vi "SubPanel_DataCollection_Rev11_v17.vi"(0 "DCPowerInformationClusterArray_Input":T1[](array[typedef]), 1 "VISAPowerInfoInputArray":T4[](array[typedef]), 2 "Run Data SubPanel Input":T6, 3 "RF Block Input Array":T5[](array[typedef]), 4 "Oscilloscope Configuration Input Array":T2[](array[typedef]) {"vertical coupling" items=["AC", "DC", "Ground"]}, 5 "Plot Color Array":u32[](array[colorbox])=[16711686, 65351, 8978420, 14474240, 16139007, 16752640, 8958719, 16758973, 16777215, 46792, 11992992, 12961221, 16763690, 12600063, 16711835, 2953983, 40796, 13111296, 13352613, 9221011, 12964076, 12819897, 65442, 16776704, 14540253, 16740729, 10658047, 10813344, 16753521, 13413843, 8691115, 10339240, 14401205, 16746704, 7467519, 16775978, 13872558, 11387603, 13354405, 10420227, 13107364, 4060, 35208, 11817216, 7566080, 40796, 7539456, 2837073, 6372186, 7499083, 10648702, 16757152], 6 "New Run?":bool, 7 "error in":errorcluster) -> (20 "DCPowerInformationClusterArray_Output":T1[](array[typedef]), 21 "VISAPowerInfoOutputArray":T4[](array[typedef]), 22 "Run Data SubPanel Output":T6, 23 "RF Subpanel Output":T5[](array[typedef]), 24 "Oscilloscope Info Array":T7(array[cluster]) {"vertical coupling" items=["AC", "DC", "Ground"]}, 25 "Reinitialize?":bool, 26 "Data Was Collected?":bool, 27 "error out":errorcluster)   [LabVIEW 2019]
uses:
  Controls/DataBlockControl.ctl
  Controls/RFBlockControl.ctl
  <instrlib>/niScope/Controls/niScope vertical coupling.ctl
  Controls/VISA_power_Control.ctl
  Controls/OscilloscopeBlockControl2.ctl
  Controls/DCPowerBlock_byInstrument_Control.ctl
  Controls/QueueDataControl_V3.ctl
  <instrlib>/niDMM/nidmm.llb/niDMM Trigger.ctl
  <instrlib>/niDMM/nidmm.llb/niDMM Resolution in Digits.ctl
  <instrlib>/niDMM/nidmm.llb/niDMM Function.ctl
  <instrlib>/niScope/Acquire/Fetch/niScope Multi Fetch Binary 16.vi
  <instrlib>/niDMM/nidmm.llb/niDMM Configure Measurement Digits.vi
  <vilib>/Utility/file.llb/Write Delimited Spreadsheet (string).vi
panel:
  out "error IO":errorcluster
  in  "Software Mitigation?":bool
  in  "User Forced Reset":bool
  in  "Total Time X Min":dbl
  in  "Total Time X Max":dbl
  in  "Total Current Y Min":dbl
  in  "Total Current Y Max":dbl
  in  "Total Voltage Y Min":dbl
  in  "Total Voltage Y Max":dbl
  in  "Total Measurement Range Update":bool
  in  "Live Measurement Range Update":bool
  in  "Live Current Y Min":dbl
  in  "Live Current Y Max":dbl
  in  "Live Voltage Y Min":dbl
  in  "Live Voltage Y Max":dbl
  in  "Waveform Update":bool
  in  "Current Waveform Y Max":dbl
  in  "Current Waveform Y Min":dbl
  in  "Voltage Waveform Y Min":dbl
  in  "Voltage Waveform Y Max":dbl
  in  "Max Range 7":dbl
  in  "Min Range 7":dbl
  in  "Min Range 6":dbl
  in  "Max Range 6":dbl
  in  "Max Range 5":dbl
  in  "Min Range 5":dbl
  in  "Max Range 4":dbl
  in  "Min Range 4":dbl
  in  "Min Range 3":dbl
  in  "Max Range 3":dbl
  in  "Min Range 2":dbl
  in  "Max Range 2":dbl
  in  "Min Range 0":dbl
  in  "Min Range 1":dbl
  in  "Max Range 1":dbl
  in  "Max Range 0":dbl
  in  "Oscope Range Update":bool
  out "Oscilloscope Configuration":T2 {"vertical coupling" items=["AC", "DC", "Ground"]}
  in  "Reset Value":i32=51
  out "Pryor's Graph":dbl[][](graph)
  in  "Reset Value 2":i32=251
  out "Channel Graph 0":dbl[](graph)
  out "Channel Graph 1":dbl[](graph)
  out "Channel Graph 2":dbl[](graph)
  out "Channel Graph 3":dbl[](graph)
  out "Channel Graph 7":dbl[](graph)
  out "Channel Graph 6":dbl[](graph)
  out "Channel Graph 5":dbl[](graph)
  out "Channel Graph 4":dbl[](graph)
  out "Measurement":dbl caption="BEAM STATE (NOT ~0 IF ON)" format="%.5f"
  in  "Time showing on Live Measurements":i32=251
  in  "Device Powered?":bool=TRUE
  out "Current Measurements Live":cluster{dbl[], dbl[]}[](graph)
  out "Voltage Measurements Live":cluster{dbl[], dbl[]}[](graph)
  out "Voltage Waveform Array":waveform(dbl)[](graph)
  out "Current Waveform Array":waveform(dbl)[](graph)
  out "Current Measurements Total":cluster{dbl[], dbl[]}[](graph)
  out "Voltage Measurements Total":cluster{dbl[], dbl[]}[](graph)
  out "Exiting":bool
  out "Full Run Information":string
  out "Ready For Next Run?":bool
  in  "Next Run":bool
  out "Recording Data":bool
  in  "Record Data Toggle":bool
  out "error of collection":errorcluster
  in  "force exit SubVI":bool
  out "RF Block Parameters Output":T5
  out "RFSourceInfoArray":string[][](array[string])
  out "OscilloscopeInfoArray":string[][](array[string])
  out "DCPowerInfoArray":string[][](array[string])
  # "Background information (Important)\nThere are three sets of voltage/current graphs\n\nOne is live always and just shows what all the channels look like _______ Waveform Array\n\nOne is live when measuring and shows some duration of the recording _______ Measurements Live\n\nOne shows the entire duration of the run, but it will take a few seconds to compile, just be patient it will populate\n\n\nInstructions (More Important)"
  # "CURRENTLY CAN ONLY USE ONE OSCOPE AT A TIME"
  # "off"
  # "on"
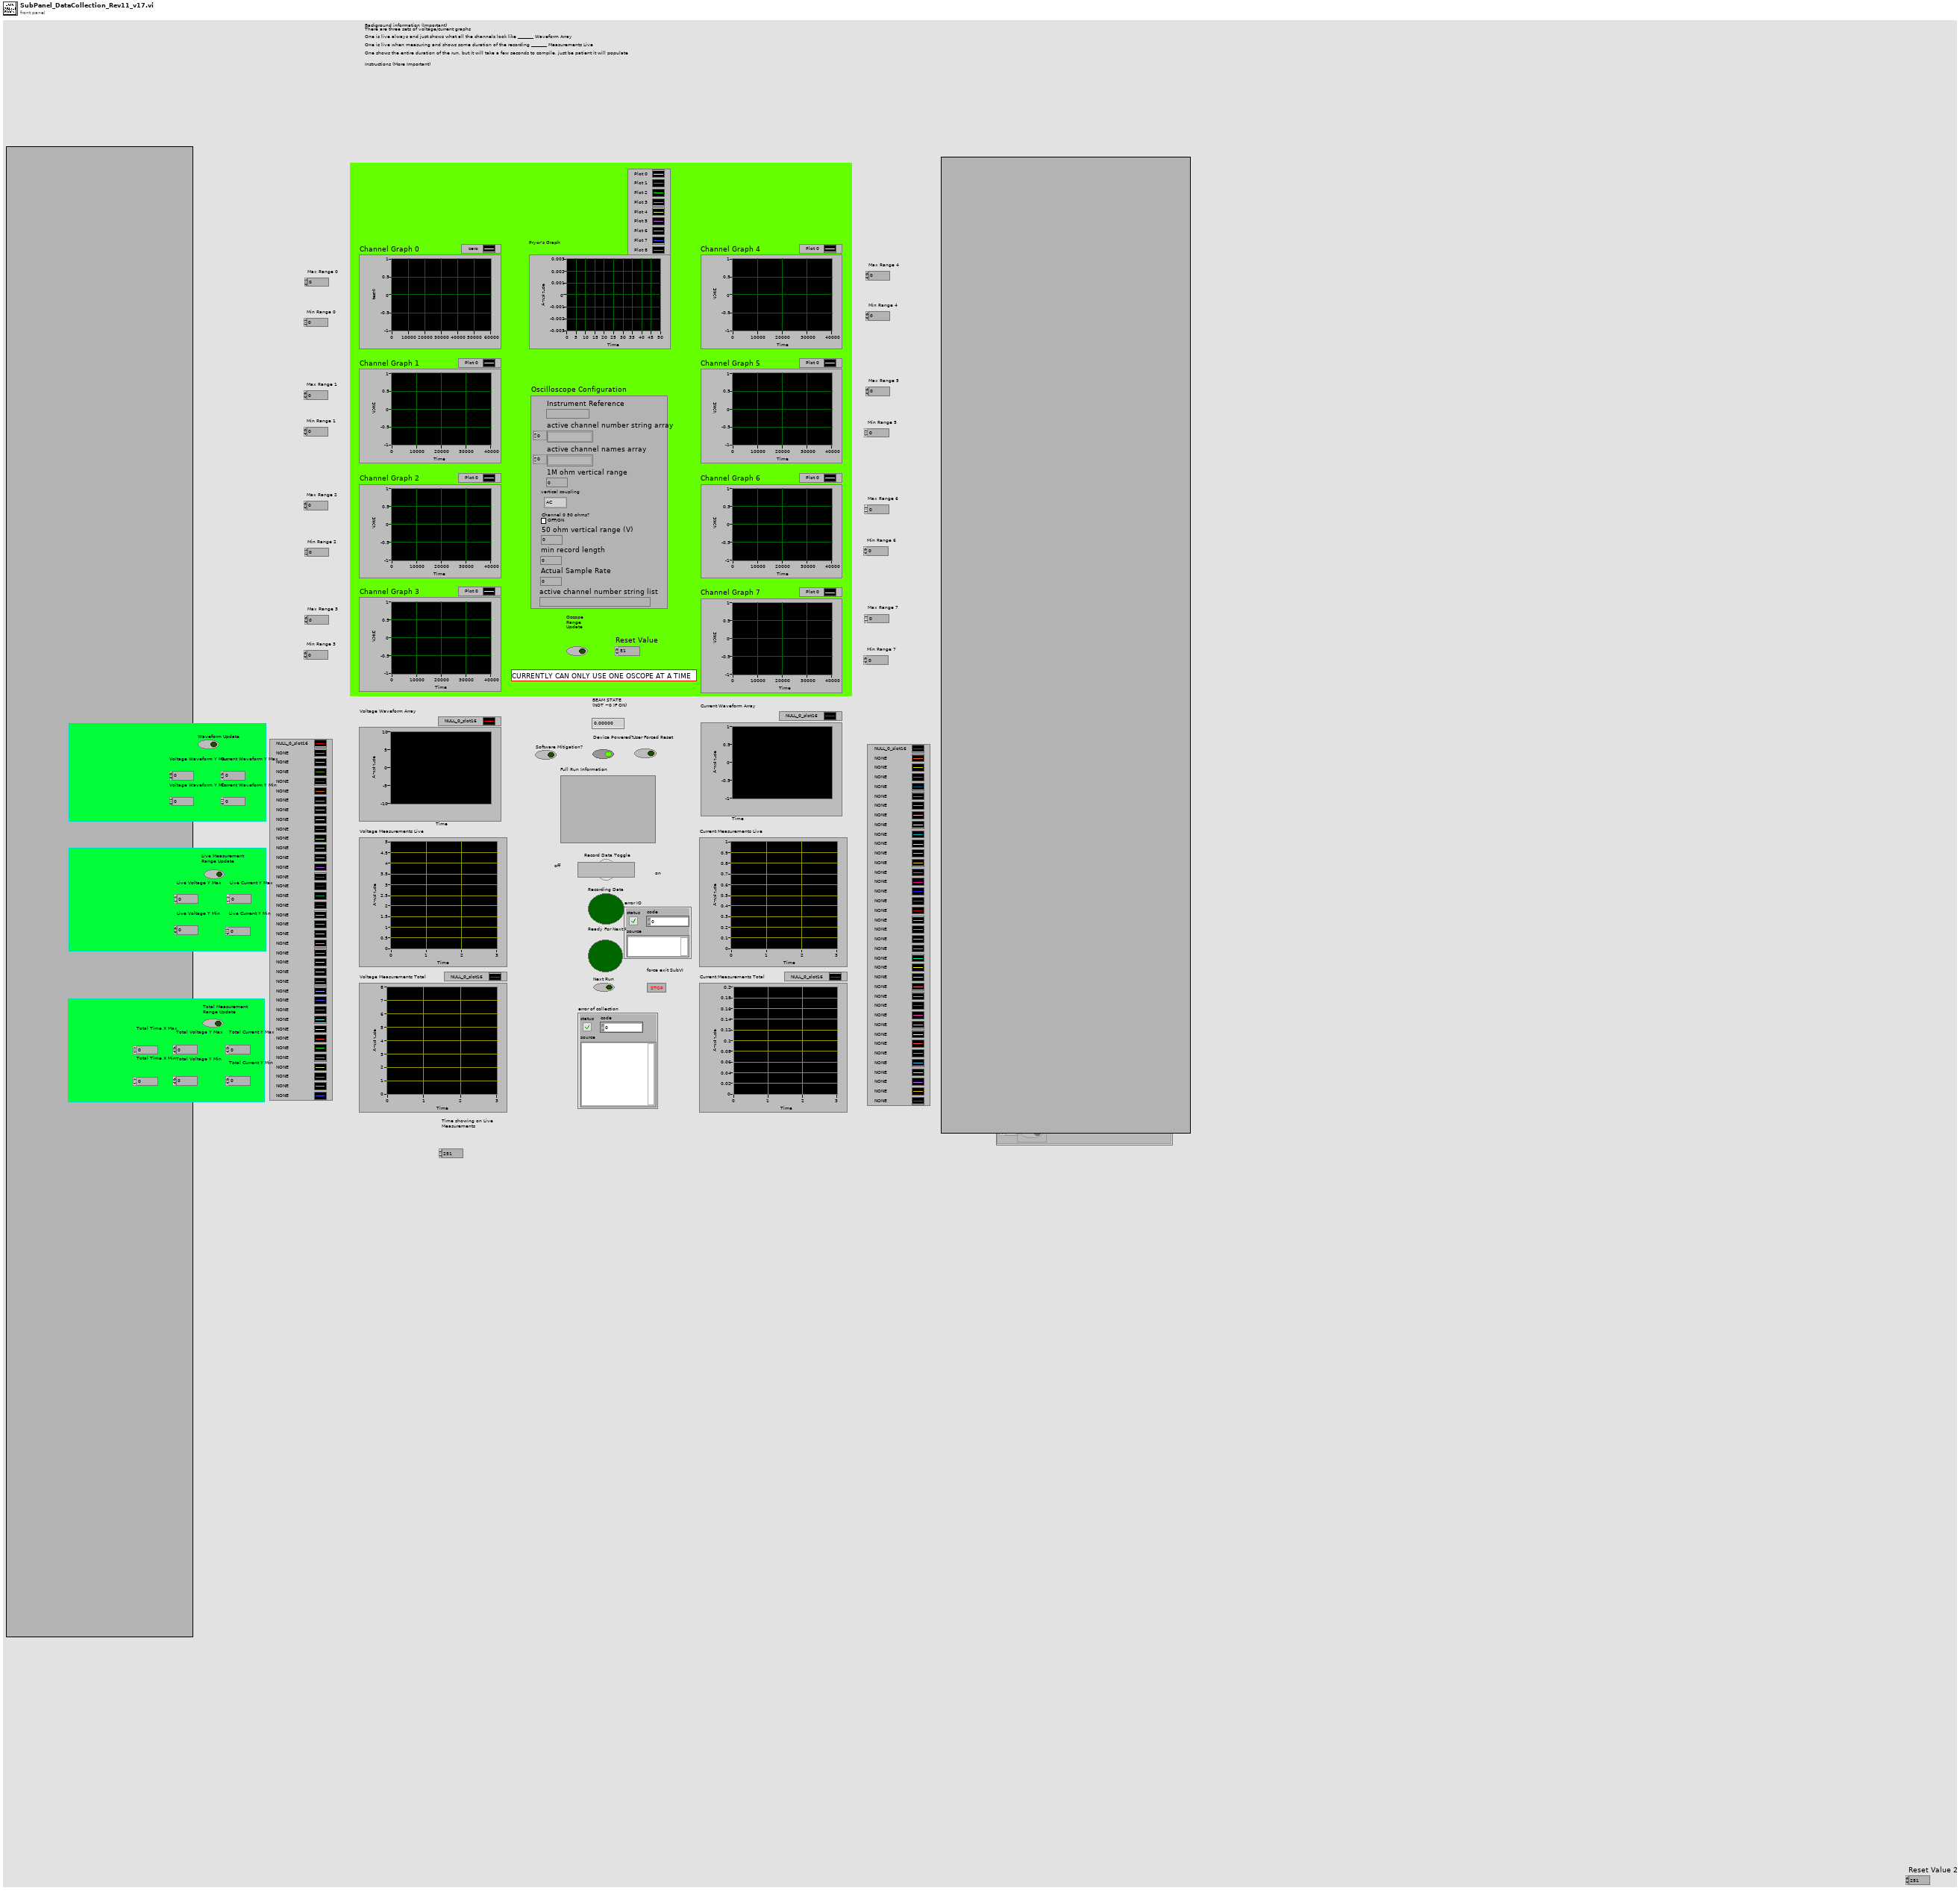
[diagram p1: front panel]
types:
  T1 = typedef "DCPowerBlock_byInstrument_Control.ctl" = cluster{"IVI Refnum out":refnum<k15>, "Active Channel Numbers String List":string, "Active Channel Numbers Array":string[], "Active Channel Voltage Array":dbl[], "Active Channel Names Array":string[], "Active Channel Current Limit Array":dbl[], "Active Channel Measure Record Delta Time Array":dbl[], "All Channel Numbers Array":string[], "Current Threshold Reset Value Array":dbl[], "Mitigation channel":bool[]}
  T2 = typedef "OscilloscopeBlockControl2.ctl" = cluster{"Instrument Reference":refnum<k15>, "active channel number string array":string[], "active channel names array":string[], "1M ohm vertical range":dbl, "vertical coupling":T3, "Channel 0 50 ohms?":bool, "50 ohm vertical range (V)":dbl, "min record length":i32, "Actual Sample Rate":dbl, "active channel number string list":string}
  T3 = typedef "niScope vertical coupling.ctl" = i32
  T4 = typedef "VISA_power_Control.ctl" = cluster{"VISA resource name":refnum<visa-resource-name>, "Active Channel List":string, "Active Channel Array":string[], "Input Array (Voltage,Current_Limit)":dbl[], "Input Array (Voltage,Current_Limit)":dbl[], "Channel Names":string[], "read buffer":string, "Channel Names Array":string[]}
  T5 = typedef "RFBlockControl.ctl" = cluster{"VISA resource name":refnum<visa-resource-name>, "RF Power State In":bool, "Frequency (GHz) Output":dbl, "Power (dBm) Output":dbl, "Instrument Name":string}
  T6 = typedef "DataBlockControl.ctl" = cluster{"Run Folder Parent Directory":path, "DUT":string, "Ion (ex Kr)":string, "Board Number":string, "Effective LET":string, "Test Type":enum16{"Single Event Latchup", "Single Event Transient", "Single Event Upset"}}
  T7 = cluster{"instrument handle out":refnum<k15>, string[], string[], "vertical range":dbl, "vertical coupling":T3, "Channel 0 50 ohms?":bool, "50 ohm vertical range (V)":dbl, "min record length":i32, "Actual Sample Rate":dbl, "channel names list":string}[]
  T8 = enum16{"open", "replace", "create", "open or create", "replace or create", "replace or create with confirmation"}
  T9 = cluster{"Array":dbl[], "Array":dbl[], "Array":dbl[], "Array":dbl[], "Array":dbl[], "Array":dbl[], "Array":dbl[], "Array":dbl[]}
  T10 = cluster{"wfm info":cluster{"actualSamples":i32, "absoluteInitialX":dbl, "relativeInitialX":dbl, "xIncrement":dbl, "offset":dbl, "gain":dbl, "reserved1":dbl, "reserved2":dbl}[], "wfm":i16[][]}
  T11 = typedef "niDMM Function.ctl" = enum16{"DC Volts", "AC Volts", "DC Current", "AC Current", "2-wire Resistance", "4-wire Resistance", "Diode", "Frequency", "Period", "AC Volts DC Coupled", "Capacitance", "Inductance", "Temperature"}
  T12 = typedef "niDMM Resolution in Digits.ctl" = dbl
  T13 = typedef "niDMM Trigger.ctl" = enum16{"Immediate", "External", "TTL 0", "TTL 1", "TTL 2", "TTL 3", "TTL 4", "TTL 5", "TTL 6", "Software", "TTL 7", "PXI Star", "LBR Trig 1", "Aux Trig 1"}
  T14 = cluster{"appended path":path, "refnum out":refnum<file>, "refnum out":refnum<file>, "refnum out":refnum<file>}
  T15 = typedef "QueueDataControl_V3.ctl" = cluster{"Array of fetched data":dbl[][][], "Channel Names Array":string[], "Voltage Waveform Array":waveform(dbl)[], "Current Waveform Array":waveform(dbl)[], "Resetting Time":timestamp, "Beam Logic":dbl}
  T16 = cluster{"IVI Refnum out":refnum<k15>, string, "voltage level channel 23":dbl, "Channel Name 23":string, "Current Limit":dbl, "Measure Record dt":dbl, string, "Current Threshold Reset Value Array":dbl, "Mitigation Channel":bool}[]
  T17 = cluster{"created path":path, refnum<file>[], refnum<file>[]}
  T18 = cluster{"created path":path, "DCPowerInformationArrayOutput_byChannel":cluster{"IVI Refnum out":refnum<k15>, string, "voltage level channel 23":dbl, "Channel Name 23":string, "Current Limit":dbl, "Measure Record dt":dbl, string, "Current Threshold Reset Value Array":dbl, "Mitigation Channel":bool}[], string[]}
  T19 = cluster{"actualSamples":i32, "absoluteInitialX":dbl, "relativeInitialX":dbl, "xIncrement":dbl, "offset":dbl, "gain":dbl, "reserved1":dbl, "reserved2":dbl}[]
  T20 = enum16{"big-endian, network order", "native, host order", "little-endian"}
  T21 = cluster{"Array of fetched data":dbl[][], string, i32[]}
  T22 = enum16{"Single Event Latchup", "Single Event Transient", "Single Event Upset"}
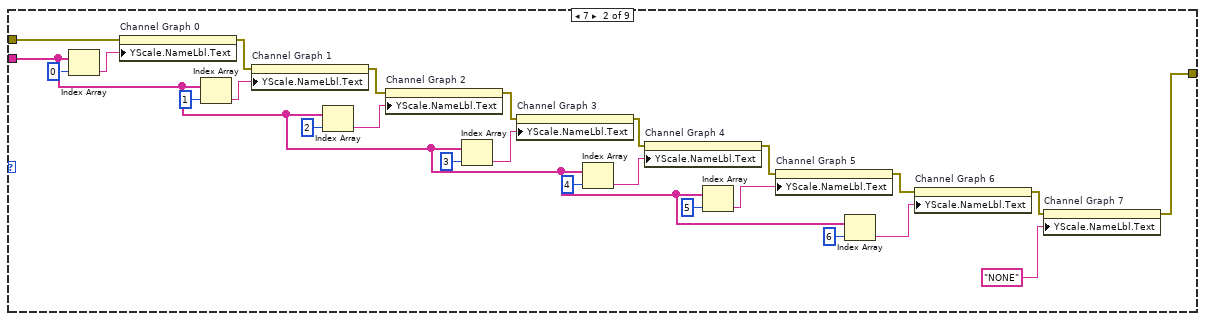
[diagram p2: hidden frame]
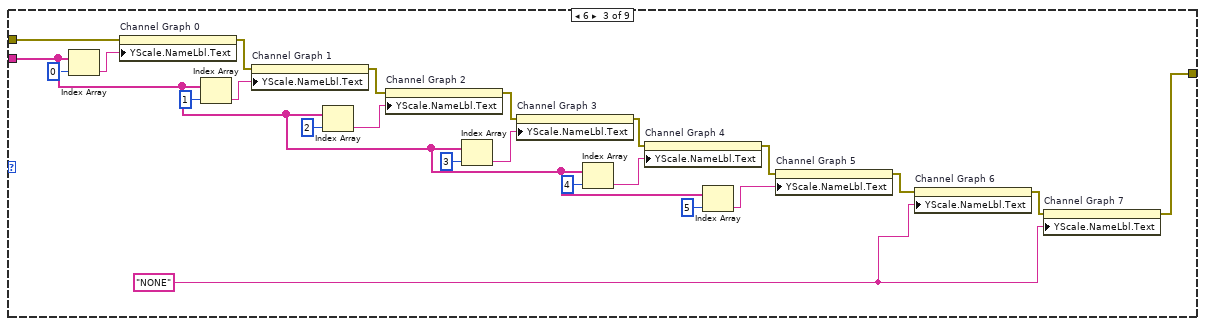
[diagram p3: hidden frame]
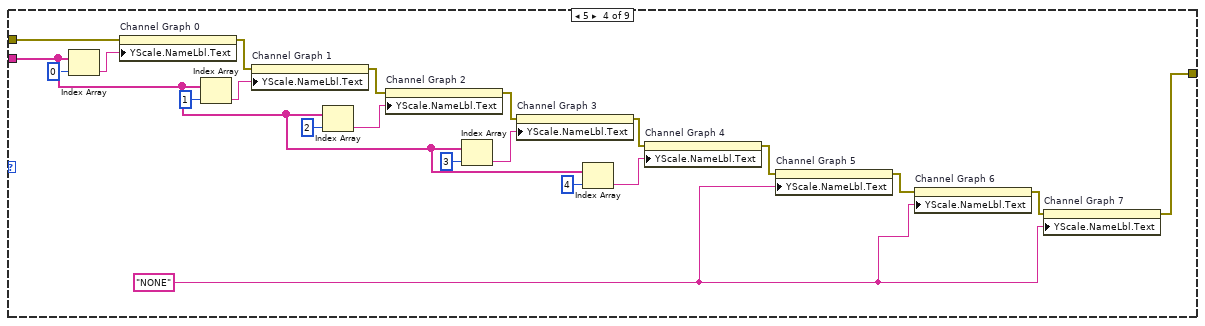
[diagram p4: hidden frame]
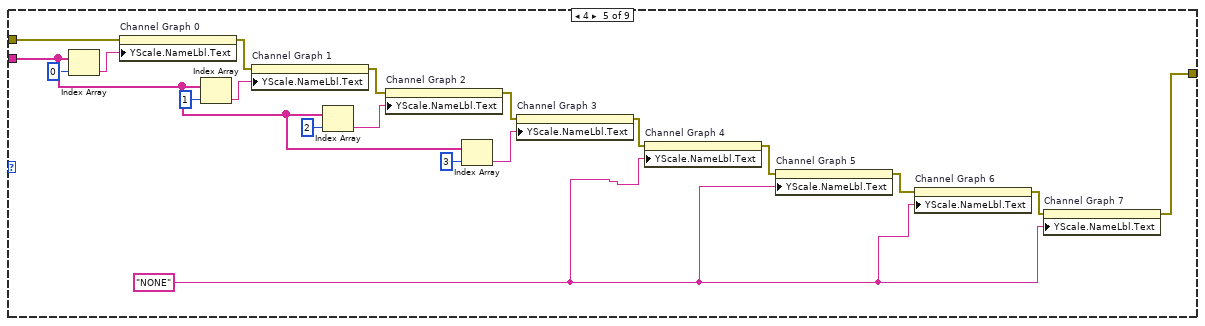
[diagram p5: hidden frame]
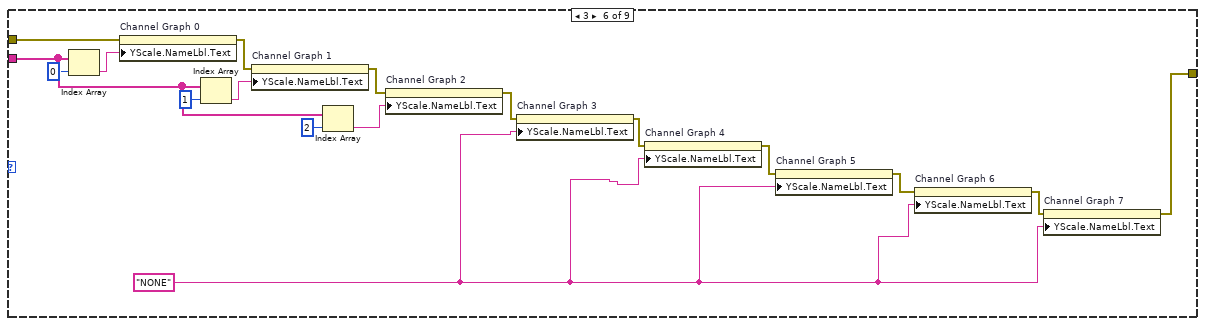
[diagram p6: hidden frame]
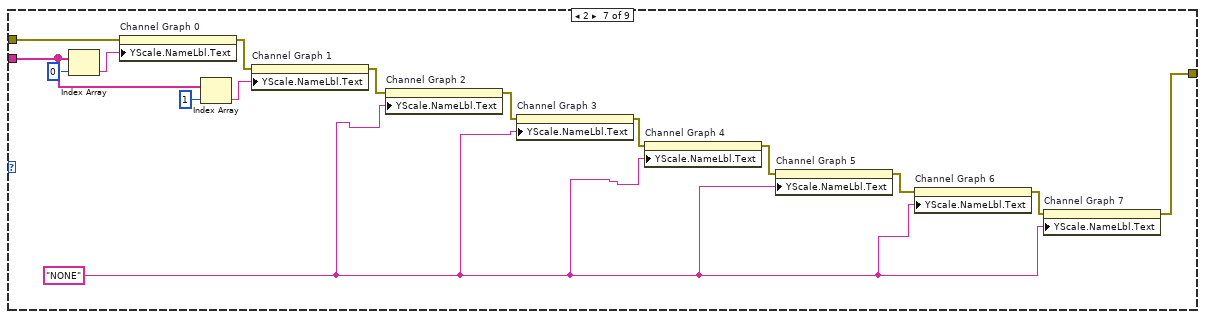
[diagram p7: hidden frame]
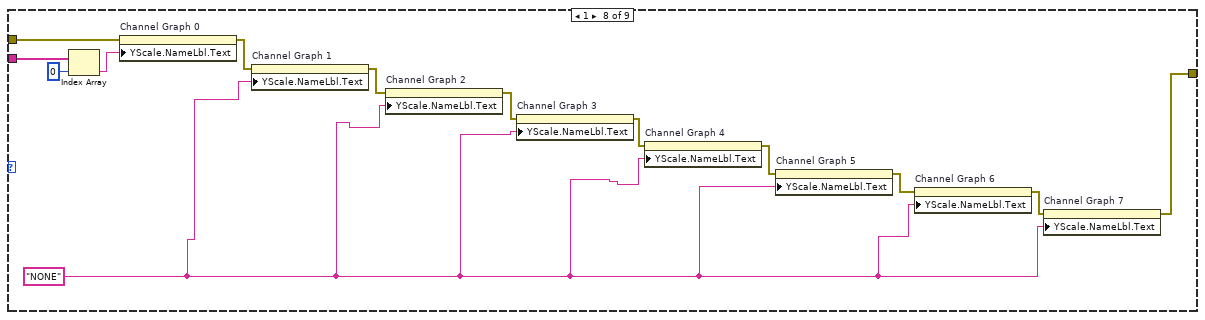
[diagram p8: hidden frame]
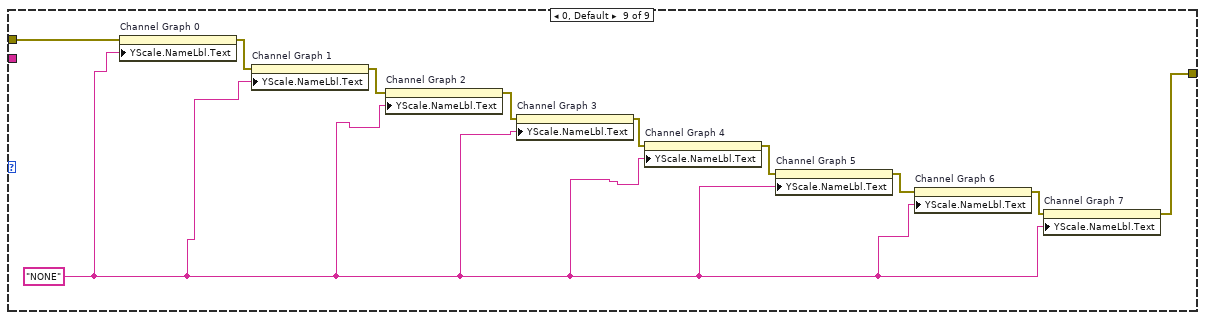
[diagram p9: hidden frame]
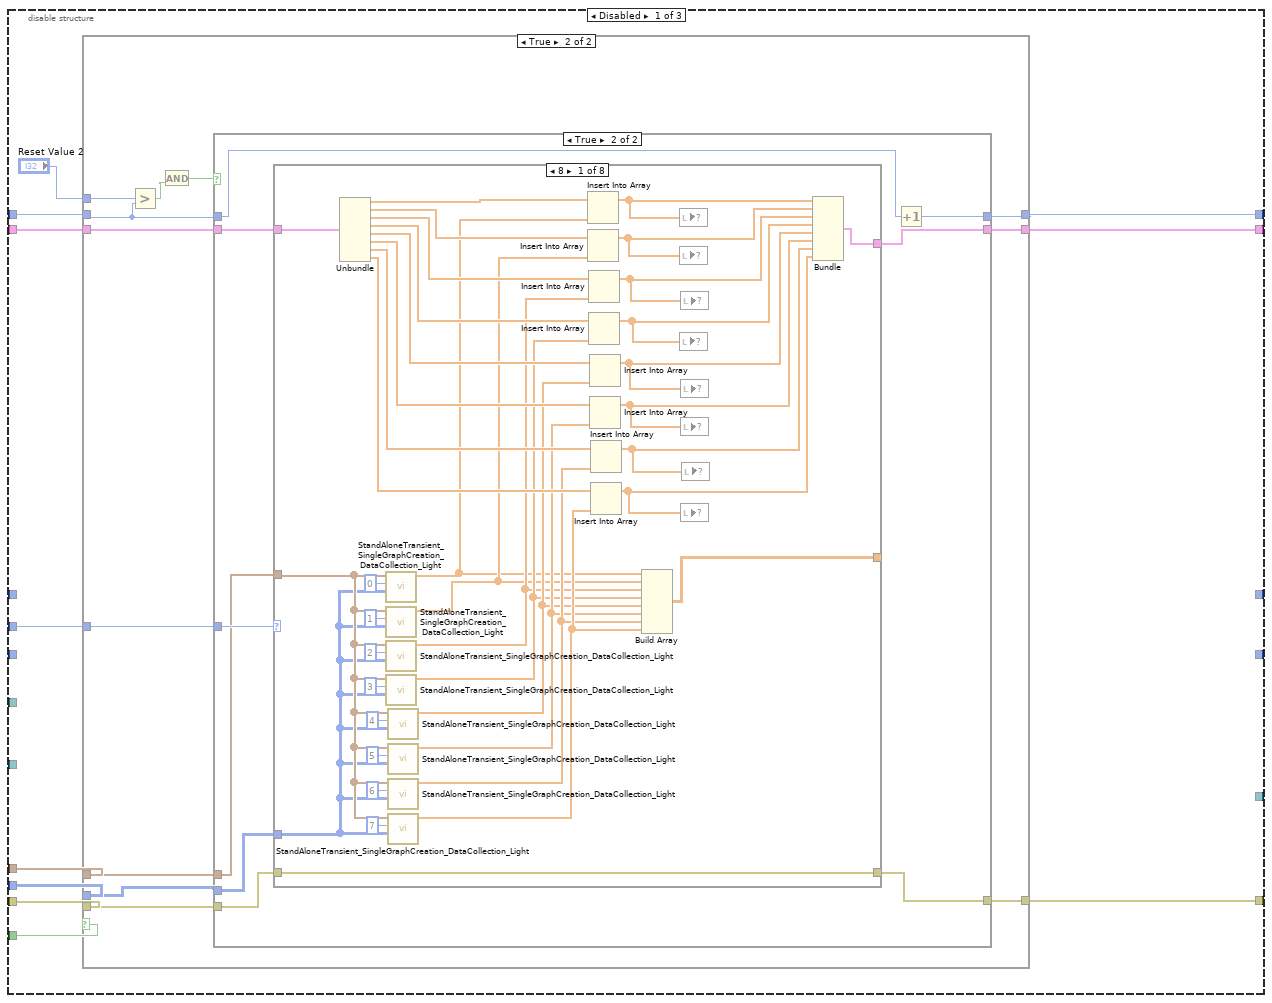
[diagram p10: hidden frame]
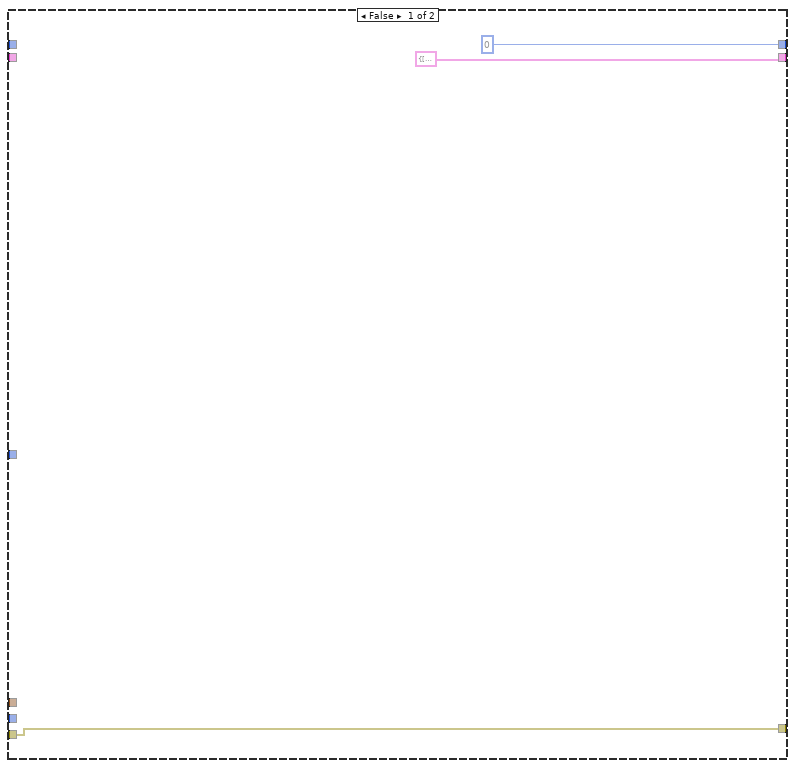
[diagram p12: hidden frame]
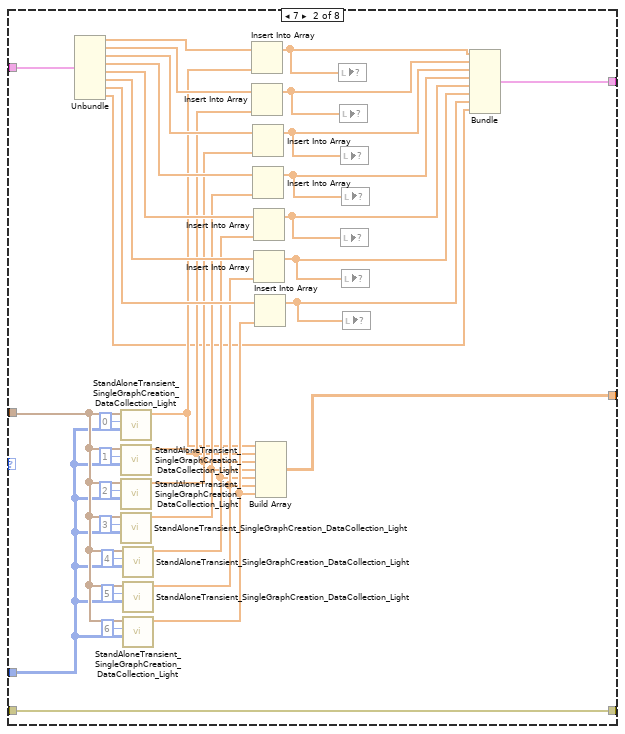
[diagram p13: hidden frame]
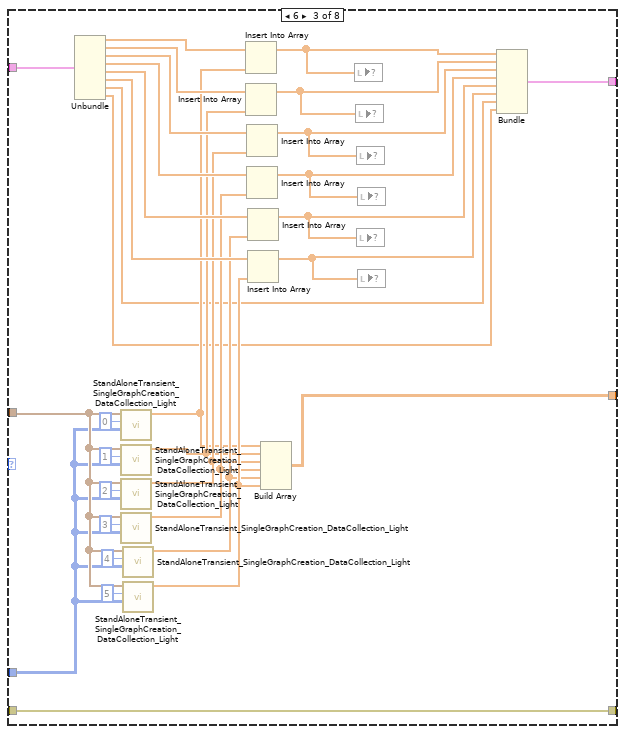
[diagram p14: hidden frame]
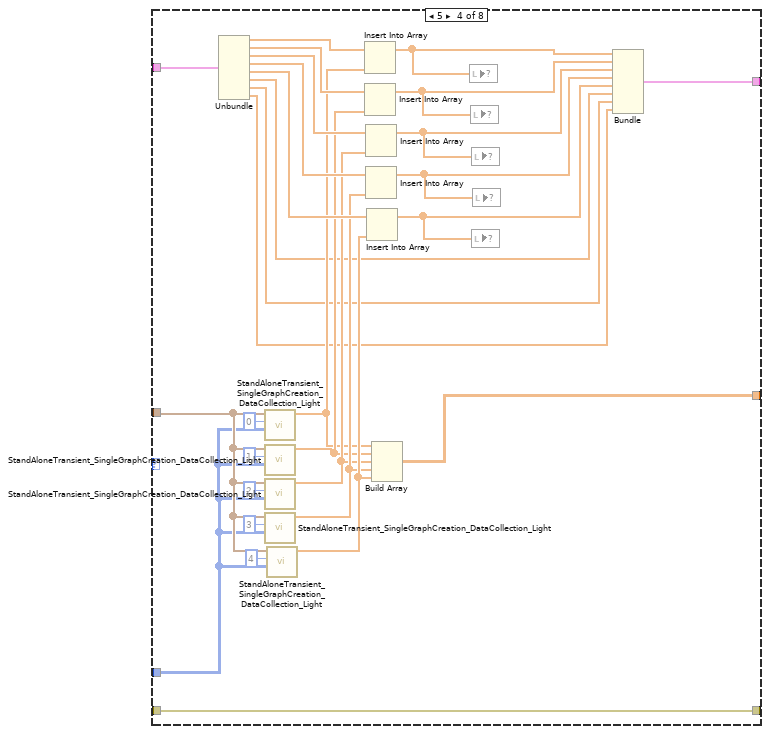
[diagram p15: hidden frame]
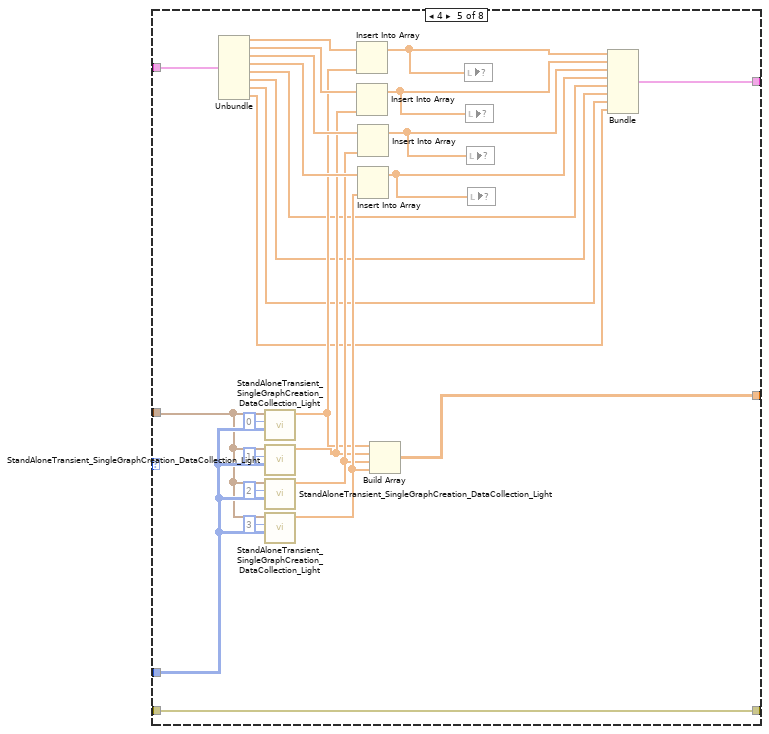
[diagram p16: hidden frame]
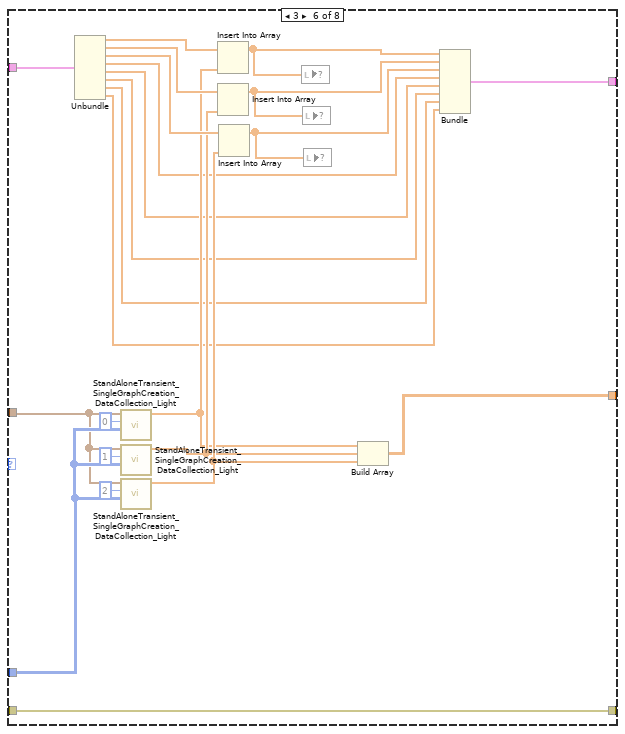
[diagram p17: hidden frame]
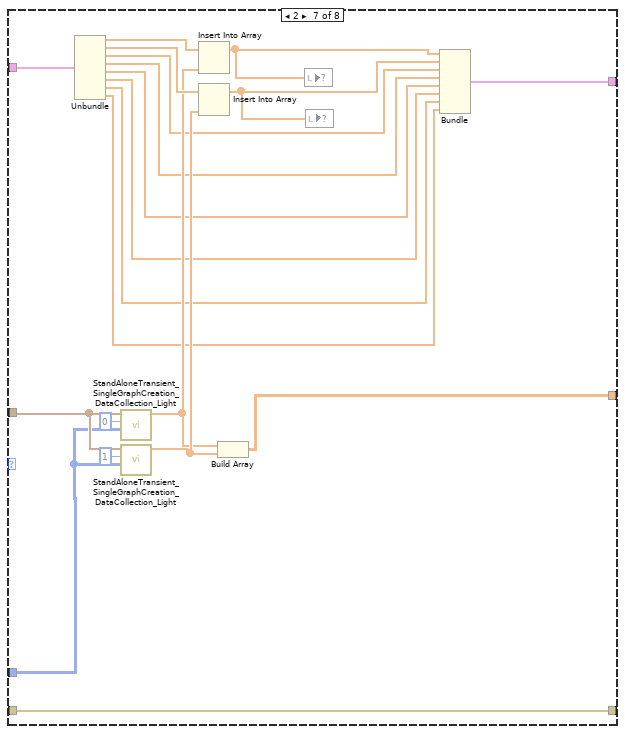
[diagram p18: hidden frame]
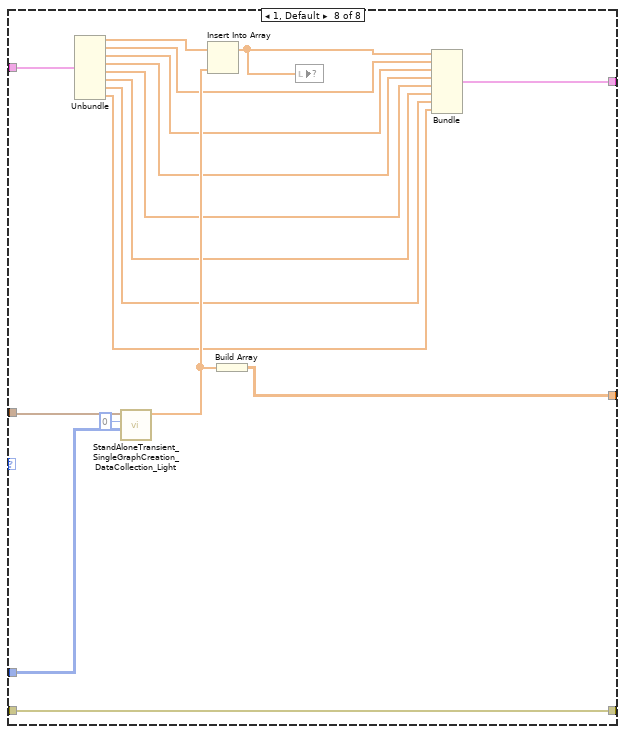
[diagram p19: hidden frame]
diagram:
  w39 = 1
  w67 = T12 3.5 items=["3 1/2"=3.5, "4 1/2"=4.5, "5 1/2"=5.5, "6 1/2"=6.5, "7 1/2"=7.5] ("Resolution in Digits")
  w82 = cluster{dbl[], dbl[]}[] [] ("array")
  (unwired) timestamp(0 s since 1904-01-01) ("seconds since 1Jan1904")
  (unwired) 10000 ("binary file indexor in")
  (unwired) 0
  (unwired) 0 ("x")
  (unwired) errorcluster {"status"=FALSE, "code"=0, "source"=""} ("error out")
  (unwired) T14 {"appended path"=path "", "refnum out"=refnum, "refnum out"=refnum, "refnum out"=refnum} ("BinaryRefObjects")
  (unwired) string[] ["Instrument Name", "Channel Name", "Instrument Channel Number", "Voltage (V)", "Current Limit (A)", "Measure Record delta Time (s)"] ("new element/subarray")
  w161 = T15 {"Array of fetched data"=[], "Channel Names Array"=[], "Voltage Waveform Array"=[], "Current Waveform Array"=[], "Resetting Time"=timestamp(0 s since 1904-01-01), "Beam Logic"=0.0} ("DCPower Queue Data Double Array Format")
  (unwired) T15 {"Array of fetched data"=[], "Channel Names Array"=[], "Voltage Waveform Array"=[], "Current Waveform Array"=[], "Resetting Time"=timestamp(0 s since 1904-01-01), "Beam Logic"=0.0} ("DCPower Double Array Queue")
  (unwired) T6 {"Run Folder Parent Directory"=path "", "DUT"="", "Ion (ex Kr)"="", "Board Number"="", "Effective LET"="", "Test Type"=enum."Single Event Latchup"} ("Run Data Configuration")
  # "A flag to state if the devices are powered on or off"
  # "Need to make a function that will decrease the amount of loops if there are more channels active. Just exponential decay or a X/Y function but need some kind of offset which will probably be experimentally determined"
  # "Reset the graph that is saving every 10 seconds of data. Every reset the low bound of the ten seconds is"
  # "Indicator if the system is ready for another run. Also indicates if data was actually collected"
  # "Resets the system to start recording"
  # "A flag to ensure the START A NEW DATACOLLECTION RUN  warning message shows only once and doesn't lock the system"
  # "Initiating the queue"
  # "echoing run information"
  # "Checking if this is a new run. If it is, a new folder is created along with references to a datafile node. If it is not new (i.e. you didn't start recording data because you needed to make a last minute change and pressed forced exit subvi), the previous folder that is theoretically empty (or just has the .txt files is used"
  # "If yes, you go into this subVI"
  # "This is the message at the beginning confirming if you want to make small changes to the program (i.e. LET)"
  # "Parameters from the configuration stage of this program"
  # "Need to change to reflect number of channels that are being recorded. Collect this from a parameters file eventually that will be created"
  # "Initiating all of the DC Power instruments (doing this here so because we force abort channels in the DCPower setup because buffer overflow issues. Iterating over the instrument array and the active channel list"
  n1 = flat-sequence {
    tunnel: [w180] -> w165
    tunnel: "error in" -> [w170]
    tunnel: [w184] -> w166
    tunnel: "Run Data SubPanel Input" -> [w172]
    frame #0 {
      n2 = disable-structure shown="Enabled" {
        disable-tunnel: w170 -> [w187 w198]
        disable-tunnel: [w196 w198] -> w169
        frame Enabled {
          n3 = property on="Voltage Measurements Live" class="XYGraph (strict)"(error in=w187, "BG Color"=u32 0 ("Plot.Plot Color"), "Plot.Plot Interpolation"=u8 2) -> (error out=w186:errorcluster)  [unwired: 1 in, 1 out]
          n4 = property on="Current Measurements Live" class="XYGraph (strict)"(error in=w186, "BG Color"=u32 0 ("Plot.Plot Color"), "Plot.Plot Interpolation"=u8 2) -> (error out=w185:errorcluster)  [unwired: 1 in, 1 out]
          n5 = property on="Voltage Measurements Total" class="XYGraph (strict)"(error in=w185, "BG Color"=u32 0 ("Plot.Plot Color"), "Plot.Plot Interpolation"=u8 2) -> (error out=w197:errorcluster)  [unwired: 1 in, 1 out]
          n6 = property on="Current Measurements Total" class="XYGraph (strict)"(error in=w197, "BG Color"=u32 0 ("Plot.Plot Color"), "Plot.Plot Interpolation"=u8 2) -> (error out=w196:errorcluster)  [unwired: 1 in, 1 out]
        }
        frame Disabled {
        }
      }
      n7 = local write "Voltage Measurements Total"(cluster{dbl[], dbl[]}[] [] ("Voltage Measurements")) -> ()
      n8 = local write "Current Measurements Total"(cluster{dbl[], dbl[]}[] [] ("Current Measurements")) -> ()
      n9 = local write "Recording Data"(FALSE ("Recording Data")) -> ()
      n10 = local write "Exiting"(FALSE ("Forced Exit")) -> ()
      n11 = call "Convert_RunInfoCluster_2_RunInfoStringList.vi"("error in"=w169, "Run Number"="", "Run Data SubPanel Input"=w172) -> ("error output"=w173:errorcluster, "Run Data Output"=w174:string)
      n12 = call "Display Message to User"("error in (no error)"=w173, "Enable"=TRUE, "Message"=w174) -> ("error out"=w180:errorcluster)  [unwired: 7 in, 1 out]
      n13 = Two Button Dialog(message="Changing the LET?", 1:"No" ("F button name (\"Cancel\")"), 2:"Yes" ("T button name (\"OK\")")) -> (T button?=w184:bool)
    }
  }
  n14 = call "Convert_InstrumentReferenceArray_2_ChannelReferenceArray.vi"("error in (no error)"=w165, "DCPowerInformationClusterArray_Input"="DCPowerInformationClusterArray_Input") -> ("error out"=w164:errorcluster, "DCPowerInformationArrayOutput_byChannel"=w132:T16)
  n15 = case shown="True" w166 {
    tunnel: "Run Data SubPanel Input" -> [w200 w204]
    tunnel: [w200 w203] -> w147
    tunnel: [w199 w202] -> w131
    tunnel: w164 -> [w199 w201]
    frame False {
    }
    frame True {
      n16 = disable-structure shown="Enabled" {
        disable-tunnel: w204 -> [w208 w210]
        disable-tunnel: [w207 w209] -> w203
        disable-tunnel: [w206 w212] -> w202
        disable-tunnel: w201 -> [w205 w211]
        frame Disabled {
          n17 = call "Change_RunInfo.vi"("error in (no error)"=w205, "Run Data SubPanel in"=w208) -> ("error out"=w206:errorcluster, "Run Data SubPanel out"=w207:T6)
        }
        frame Enabled {
          n18 = call "Change_RunInfo_V2.vi"("error in (no error)"=w211, "Run Data SubPanel in"=w210) -> ("error out"=w212:errorcluster, "Run Data SubPanel out"=w209:T6)
        }
      }
    }
  }
  n19 = Unbundle(w147) -> ("Run Folder Parent Directory"=w115:path)  [unwired: 5 out]
  n20 = call "Determining_Change_RunNumber.vi"("error in"=w131, "Run Folder Parent Directory"=w115) -> ("error out"=w124:errorcluster, "Array"=w125:dbl[], "String"=w126:string, "path out"=w127:path, "Proposed Run Number"=w123:i32, "T button?"=w128:bool)  [unwired: 4 in]
  n21 = call "Change_RunNumber.vi"("Valid Run Number"=w123, "Changing the run number?"=w128, "error in (no error)"=w124, "Array"=w125, "String in"=w126, "path in"=w127) -> ("error out"=w130:errorcluster, "String out"=w129:string)  [unwired: 4 in]
  n22 = Concatenate Strings("Run_", w129) -> (w116:string)
  n23 = Index Array(array="Oscilloscope Configuration Input Array", index=0) -> (element=w119:T2)
  n24 = Unbundle By Name(w119) -> ("active channel number string array"=w108:string[])
  n25 = Array Size(array=w132) -> (size(s)=w57:i32)
  n26 = Array Size(array=w108) -> (size(s)=w50:i32)
  n27 = Bundle("subfolder"="DCPower", w57) -> (w111:cluster{"subfolder":string, i32})  [unwired: 1 in]
  n28 = Bundle("subfolder"="Oscilloscope", w50) -> (w110:cluster{"subfolder":string, i32})  [unwired: 1 in]
  n29 = Build Array(w111, w110) -> (w107:cluster{"subfolder":string, i32}[])
  n30 = call "InitialFileFolderCreation_V2.vi"("New Run?"="New Run?", "error in (no error)"=w130, "Run Number"=w116, "Subfolders&NumChannelsRecorded"=w107, "base path"=w115) -> ("error out"=w109:errorcluster, "SupplementalDataFileReferenceObjectArrayWsubfolders"=w100:refnum<file>[][], "DataFileReferenceObjectArrayWsubfolders"=w101:refnum<file>[][], "created path array"=w103:path[])  [unwired: 3 in]
  n31 = Index Array(array=w100, index (row)=0) -> (element=w59:refnum<file>[])  [unwired: 1 in]
  n32 = Index Array(array=w103, index=0) -> (element=w8:path)
  n33 = Index Array(array=w101, index (row)=1) -> (element=w56:refnum<file>[])  [unwired: 1 in]
  n34 = Index Array(array=w100, index (row)=1) -> (element=w52:refnum<file>[])  [unwired: 1 in]
  n35 = Index Array(array=w103, index=1) -> (element=w97:path)
  n36 = Index Array(array=w101, index (row)=0) -> (element=w63:refnum<file>[])  [unwired: 1 in]
  n37 = Array Subset(array=w63, index=0, length=w57) -> (w61:refnum<file>[])
  n38 = Array Subset(array=w56, index=0, length=w50) -> (w55:refnum<file>[])
  n39 = Array Subset(array=w59, index=0, length=w57) -> (w58:refnum<file>[])
  n40 = Array Subset(array=w52, index=0, length=w50) -> (w51:refnum<file>[])
  n41 = Bundle("created path"=w97, w55, w51) -> (w114:T17)  [unwired: 1 in]
  n42 = call "Convert_RunInfoCluster_2_RunInfoStringList.vi"("error in"=w109, "Run Number"=w116, "Run Data SubPanel Input"=w147) -> ("error output"=w146:errorcluster, "Run Data Output"=→"Full Run Information":string)
  n43 = for {
    shift-right: [w214] -> w139
    shift-left: w146 -> [w215]
    tunnel: "DCPowerInformationClusterArray_Input" -> [w217] mode=indexing
    n44 = Unbundle(w217) -> ("IVI Refnum out"=w213:refnum<k15>, "Active Channel Numbers String List"=w216:string)  [unwired: 8 out]
    n45 = call <instrlib>:"niDCPower Initiate With Channels.vi"("error in (no error)"=w215, "channel name"=w216, "instrument handle"=w213) -> ("error out"=w214:errorcluster)  [unwired: 7 in, 1 out]
  }
  n46 = disable-structure shown="Enabled" {
    disable-tunnel: "Plot Color Array" -> [w220 _]
    disable-tunnel: [w219 w226] -> w140
    disable-tunnel: w139 -> [w218 w226]
    frame Disabled {
      n47 = for {
        shift-right: [w223] -> w219
        shift-left: w218 -> [w225]
        tunnel: w220 -> [_] mode=indexing
        i -> [w221]
        w222 = "NONE" ("Plot.Plot Name")
        n48 = property on="Current Measurements Live" class="XYGraph (strict)"(error in=w225, "Active Plot"=w221, "Plot.Plot Name"=w222) -> (error out=w224:errorcluster)  [unwired: 1 in, 1 out]
        n49 = property on="Voltage Measurements Live" class="XYGraph (strict)"(error in=w224, "Active Plot"=w221, "Plot.Plot Name"=w222) -> (error out=w223:errorcluster)  [unwired: 1 in, 1 out]
      }
    }
    frame Enabled {
    }
  }
  n50 = case shown="No Error" w140 {
    selector: w140 -> [w227 _]
    tunnel: [w227 w228] -> w134
    tunnel: w139 -> [_ w228]
    frame No Error {
    }
    frame Error {
    }
  }
  n51 = disable-structure shown="Enabled" {
    disable-tunnel: [w235 w295] -> w142
    disable-tunnel: w132 -> [w234 w296]
    disable-tunnel: "Plot Color Array" -> [w229 _]
    disable-tunnel: [w233 w294] -> w135
    disable-tunnel: w134 -> [w231 w294]
    frame Enabled {
      n52 = for {
        tunnel: w229 -> [_] mode=indexing
        shift-right: [w251] -> w232
        shift-left: w231 -> [w249]
        i -> [w250]
        w252 = "NONE" ("Plot.Plot Name")
        n53 = case shown="Error .." w249 {
          tunnel: [errorcluster {"status"=FALSE, "code"=0, "source"=""} ("error output") errorcluster {"status"=FALSE, "code"=0, "source"=""} ("error output")] -> w248
          frame No Error {
          }
          frame Error {
          }
        }
        n54 = property on="Current Waveform Array" class="WFChart (strict)"(error in=w248, "Active Plot"=w250, "Plot.Plot Name"=w252) -> (error out=w246:errorcluster)  [unwired: 1 in, 1 out]
        n55 = disable-structure shown="Disabled" {
          disable-tunnel: [w261 errorcluster {"status"=FALSE, "code"=0, "source"=""} ("error out")] -> w247
          disable-tunnel: w246 -> [w261 _]
          frame Disabled {
          }
          frame Enabled {
          }
        }
        n56 = property on="Voltage Waveform Array" class="WFChart (strict)"(error in=w247, "Active Plot"=w250, "Plot.Plot Name"=w252) -> (error out=w245:errorcluster)  [unwired: 1 in, 1 out]
        n57 = disable-structure shown="Disabled" {
          disable-tunnel: [w259 errorcluster {"status"=FALSE, "code"=0, "source"=""} ("error out")] -> w244
          disable-tunnel: w245 -> [w259 _]
          frame Disabled {
          }
          frame Enabled {
          }
        }
        n58 = property on="Current Measurements Live" class="XYGraph (strict)"(error in=w244, "Active Plot"=w250, "Plot.Plot Name"=w252) -> (error out=w243:errorcluster)  [unwired: 1 in, 1 out]
        n59 = disable-structure shown="Disabled" {
          disable-tunnel: [w257 errorcluster {"status"=FALSE, "code"=0, "source"=""} ("error out")] -> w242
          disable-tunnel: w243 -> [w257 _]
          frame Disabled {
          }
          frame Enabled {
          }
        }
        n60 = property on="Voltage Measurements Live" class="XYGraph (strict)"(error in=w242, "Active Plot"=w250, "Plot.Plot Name"=w252) -> (error out=w241:errorcluster)  [unwired: 1 in, 1 out]
        n61 = disable-structure shown="Disabled" {
          disable-tunnel: [w255 errorcluster {"status"=FALSE, "code"=0, "source"=""} ("error out")] -> w240
          disable-tunnel: w241 -> [w255 _]
          frame Disabled {
          }
          frame Enabled {
          }
        }
        n62 = property on="Voltage Measurements Total" class="XYGraph (strict)"(error in=w240, "Active Plot"=w250, "Plot.Plot Name"=w252) -> (error out=w239:errorcluster)  [unwired: 1 in, 1 out]
        n63 = disable-structure shown="Disabled" {
          disable-tunnel: [w253 errorcluster {"status"=FALSE, "code"=0, "source"=""} ("error out")] -> w238
          disable-tunnel: w239 -> [w253 _]
          frame Disabled {
          }
          frame Enabled {
          }
        }
        n64 = property on="Current Measurements Total" class="XYGraph (strict)"(error in=w238, "Active Plot"=w250, "Plot.Plot Name"=w252) -> (error out=w251:errorcluster)  [unwired: 1 in, 1 out]
      }
      n65 = case shown="No Error" w232 {
        selector: w232 -> [w236 _]
        tunnel: [w236 w237] -> w230
        tunnel: w231 -> [_ w237]
        frame No Error {
        }
        frame Error {
        }
      }
      n66 = for {
        tunnel: w234 -> [w281] mode=indexing
        tunnel: [w279] -> w235 mode=indexing
        shift-right: [w278] -> w233
        shift-left: w230 -> [w276]
        tunnel: w229 -> [w280] mode=indexing
        i -> [w277]
        # "Creating Array of Channel Names"
        n67 = case shown="Error .." w276 {
          tunnel: [errorcluster {"status"=FALSE, "code"=0, "source"=""} ("error output") errorcluster {"status"=FALSE, "code"=0, "source"=""} ("error output")] -> w275
          frame No Error {
          }
          frame Error {
          }
        }
        n68 = Unbundle(w281) -> ("Channel Name 23"=w279:string)  [unwired: 8 out]
        n69 = property on="Current Waveform Array" class="WFChart (strict)"(error in=w275, "Active Plot"=w277, "Plot.Plot Name"=w279, "Plot.Plot Color"=w280) -> (error out=w274:errorcluster)  [unwired: 1 in, 1 out]
        n70 = disable-structure shown="Disabled" {
          disable-tunnel: [w290 errorcluster {"status"=FALSE, "code"=0, "source"=""} ("error out")] -> w273
          disable-tunnel: w274 -> [w290 _]
          frame Disabled {
          }
          frame Enabled {
          }
        }
        n71 = property on="Voltage Waveform Array" class="WFChart (strict)"(error in=w273, "Active Plot"=w277, "Plot.Plot Name"=w279, "Plot.Plot Color"=w280) -> (error out=w272:errorcluster)  [unwired: 1 in, 1 out]
        n72 = disable-structure shown="Disabled" {
          disable-tunnel: [w288 errorcluster {"status"=FALSE, "code"=0, "source"=""} ("error out")] -> w271
          disable-tunnel: w272 -> [w288 _]
          frame Disabled {
          }
          frame Enabled {
          }
        }
        n73 = property on="Current Measurements Live" class="XYGraph (strict)"(error in=w271, "Active Plot"=w277, "Plot.Plot Name"=w279, "Plot.Plot Color"=w280) -> (error out=w270:errorcluster)  [unwired: 1 in, 1 out]
        n74 = disable-structure shown="Disabled" {
          disable-tunnel: [w286 errorcluster {"status"=FALSE, "code"=0, "source"=""} ("error out")] -> w269
          disable-tunnel: w270 -> [w286 _]
          frame Disabled {
          }
          frame Enabled {
          }
        }
        n75 = property on="Voltage Measurements Live" class="XYGraph (strict)"(error in=w269, "Active Plot"=w277, "Plot.Plot Name"=w279, "Plot.Plot Color"=w280) -> (error out=w268:errorcluster)  [unwired: 1 in, 1 out]
        n76 = disable-structure shown="Disabled" {
          disable-tunnel: [w284 errorcluster {"status"=FALSE, "code"=0, "source"=""} ("error out")] -> w267
          disable-tunnel: w268 -> [w284 _]
          frame Disabled {
          }
          frame Enabled {
          }
        }
        n77 = property on="Voltage Measurements Total" class="XYGraph (strict)"(error in=w267, "Active Plot"=w277, "Plot.Plot Name"=w279, "Plot.Plot Color"=w277) -> (error out=w266:errorcluster)  [unwired: 1 in, 1 out]
        n78 = disable-structure shown="Disabled" {
          disable-tunnel: [w282 errorcluster {"status"=FALSE, "code"=0, "source"=""} ("error out")] -> w265
          disable-tunnel: w266 -> [w282 _]
          frame Disabled {
          }
          frame Enabled {
          }
        }
        n79 = property on="Current Measurements Total" class="XYGraph (strict)"(error in=w265, "Active Plot"=w277, "Plot.Plot Name"=w279, "Plot.Plot Color"=w277) -> (error out=w278:errorcluster)  [unwired: 1 in, 1 out]
      }
    }
    frame Disabled {
      n80 = for {
        tunnel: w296 -> [w298] mode=indexing
        tunnel: [w297] -> w295 mode=indexing
        n81 = Unbundle(w298) -> ("Channel Name 23"=w297:string)  [unwired: 8 out]
      }
    }
  }
  n82 = disable-structure shown="Enabled" {
    disable-tunnel: [w299 errorcluster {"status"=FALSE, "code"=0, "source"=""} ("error out")] -> _
    disable-tunnel: _ -> [w299 _]
    frame Disabled {
    }
    frame Enabled {
    }
  }
  n83 = case shown="Error .." w135 {
    selector: w135 -> [w301 _]
    tunnel: [w301 w302] -> w133
    tunnel: w134 -> [_ w302]
    frame No Error {
    }
    frame Error {
    }
  }
  n84 = disable-structure shown="Enabled" {
    disable-tunnel: w133 -> [w306 w308]
    disable-tunnel: [w305 w308] -> w13
    disable-tunnel: [w304 _] -> w143
    disable-tunnel: w161 -> [w303 _]
    frame Enabled {
      n85 = Obtain Queue(name (unnamed)="DCPowerQueue", element data type=w303, error in (no error)=w306) -> (queue out=w304:refnum<queue>, error out=w305:errorcluster)  [unwired: 2 in, 1 out]
    }
    frame Disabled {
    }
  }
  n86 = Index Array(array="Oscilloscope Configuration Input Array", index=0) -> (element=w14:T2)
  "Oscilloscope Configuration" <- w14
  n87 = Unbundle By Name(w14) -> ("active channel names array"=w11:string[])
  n88 = Bundle("created path"=w8, "DCPowerInformationArrayOutput_byChannel"=w132, w142) -> (w158:T18)  [unwired: 1 in]
  n89 = Array Size(array=w142) -> (size(s)=w81:i32)
  n90 = Array Size(array=w11) -> (size(s)=w12:i32)
  n91 = case shown="8" w12 {
    tunnel: w13 -> [w327 w352 w375 w396 w415 w432 w447 w460 w470]
    tunnel: [w326 w351 w374 w395 w414 w431 w446 w459 w469] -> w3
    tunnel: w11 -> [w323 w348 w371 w392 w411 w428 w443 w457 _]
    frame 8 {
      n92 = Index Array(array=w323, index=0) -> (element=w325:string)
      n93 = property on="Channel Graph 0" class="WFGraph (strict)"(error in=w327, "YScale.NameLbl.Text"=w325) -> (error out=w334:errorcluster)  [unwired: 1 in, 1 out]
      n94 = Index Array(array=w323, index=1) -> (element=w324:string)
      n95 = property on="Channel Graph 1" class="WFGraph (strict)"(error in=w334, "YScale.NameLbl.Text"=w324) -> (error out=w333:errorcluster)  [unwired: 1 in, 1 out]
      n96 = Index Array(array=w323, index=2) -> (element=w314:string)
      n97 = property on="Channel Graph 2" class="WFGraph (strict)"(error in=w333, "YScale.NameLbl.Text"=w314) -> (error out=w332:errorcluster)  [unwired: 1 in, 1 out]
      n98 = Index Array(array=w323, index=3) -> (element=w313:string)
      n99 = property on="Channel Graph 3" class="WFGraph (strict)"(error in=w332, "YScale.NameLbl.Text"=w313) -> (error out=w331:errorcluster)  [unwired: 1 in, 1 out]
      n100 = Index Array(array=w323, index=4) -> (element=w312:string)
      n101 = property on="Channel Graph 4" class="WFGraph (strict)"(error in=w331, "YScale.NameLbl.Text"=w312) -> (error out=w330:errorcluster)  [unwired: 1 in, 1 out]
      n102 = Index Array(array=w323, index=5) -> (element=w311:string)
      n103 = property on="Channel Graph 5" class="WFGraph (strict)"(error in=w330, "YScale.NameLbl.Text"=w311) -> (error out=w329:errorcluster)  [unwired: 1 in, 1 out]
      n104 = Index Array(array=w323, index=6) -> (element=w310:string)
      n105 = property on="Channel Graph 6" class="WFGraph (strict)"(error in=w329, "YScale.NameLbl.Text"=w310) -> (error out=w328:errorcluster)  [unwired: 1 in, 1 out]
      n106 = Index Array(array=w323, index=7) -> (element=w309:string)
      n107 = property on="Channel Graph 7" class="WFGraph (strict)"(error in=w328, "YScale.NameLbl.Text"=w309) -> (error out=w326:errorcluster)  [unwired: 1 in, 1 out]
    }
    frame 7 {
      n108 = Index Array(array=w348, index=0) -> (element=w350:string)
      n109 = property on="Channel Graph 0" class="WFGraph (strict)"(error in=w352, "YScale.NameLbl.Text"=w350) -> (error out=w359:errorcluster)  [unwired: 1 in, 1 out]
      n110 = Index Array(array=w348, index=1) -> (element=w349:string)
      n111 = property on="Channel Graph 1" class="WFGraph (strict)"(error in=w359, "YScale.NameLbl.Text"=w349) -> (error out=w358:errorcluster)  [unwired: 1 in, 1 out]
      n112 = Index Array(array=w348, index=2) -> (element=w340:string)
      n113 = property on="Channel Graph 2" class="WFGraph (strict)"(error in=w358, "YScale.NameLbl.Text"=w340) -> (error out=w357:errorcluster)  [unwired: 1 in, 1 out]
      n114 = Index Array(array=w348, index=3) -> (element=w339:string)
      n115 = property on="Channel Graph 3" class="WFGraph (strict)"(error in=w357, "YScale.NameLbl.Text"=w339) -> (error out=w356:errorcluster)  [unwired: 1 in, 1 out]
      n116 = Index Array(array=w348, index=4) -> (element=w338:string)
      n117 = property on="Channel Graph 4" class="WFGraph (strict)"(error in=w356, "YScale.NameLbl.Text"=w338) -> (error out=w355:errorcluster)  [unwired: 1 in, 1 out]
      n118 = Index Array(array=w348, index=5) -> (element=w337:string)
      n119 = property on="Channel Graph 5" class="WFGraph (strict)"(error in=w355, "YScale.NameLbl.Text"=w337) -> (error out=w354:errorcluster)  [unwired: 1 in, 1 out]
      n120 = Index Array(array=w348, index=6) -> (element=w336:string)
      n121 = property on="Channel Graph 6" class="WFGraph (strict)"(error in=w354, "YScale.NameLbl.Text"=w336) -> (error out=w353:errorcluster)  [unwired: 1 in, 1 out]
      n122 = property on="Channel Graph 7" class="WFGraph (strict)"(error in=w353, "YScale.NameLbl.Text"="NONE" ("Y Scale.Name Label.Text")) -> (error out=w351:errorcluster)  [unwired: 1 in, 1 out]
    }
    frame 6 {
      w360 = "NONE" ("Y Scale.Name Label.Text")
      n123 = Index Array(array=w371, index=0) -> (element=w373:string)
      n124 = property on="Channel Graph 0" class="WFGraph (strict)"(error in=w375, "YScale.NameLbl.Text"=w373) -> (error out=w382:errorcluster)  [unwired: 1 in, 1 out]
      n125 = Index Array(array=w371, index=1) -> (element=w372:string)
      n126 = property on="Channel Graph 1" class="WFGraph (strict)"(error in=w382, "YScale.NameLbl.Text"=w372) -> (error out=w381:errorcluster)  [unwired: 1 in, 1 out]
      n127 = Index Array(array=w371, index=2) -> (element=w364:string)
      n128 = property on="Channel Graph 2" class="WFGraph (strict)"(error in=w381, "YScale.NameLbl.Text"=w364) -> (error out=w380:errorcluster)  [unwired: 1 in, 1 out]
      n129 = Index Array(array=w371, index=3) -> (element=w363:string)
      n130 = property on="Channel Graph 3" class="WFGraph (strict)"(error in=w380, "YScale.NameLbl.Text"=w363) -> (error out=w379:errorcluster)  [unwired: 1 in, 1 out]
      n131 = Index Array(array=w371, index=4) -> (element=w362:string)
      n132 = property on="Channel Graph 4" class="WFGraph (strict)"(error in=w379, "YScale.NameLbl.Text"=w362) -> (error out=w378:errorcluster)  [unwired: 1 in, 1 out]
      n133 = Index Array(array=w371, index=5) -> (element=w361:string)
      n134 = property on="Channel Graph 5" class="WFGraph (strict)"(error in=w378, "YScale.NameLbl.Text"=w361) -> (error out=w377:errorcluster)  [unwired: 1 in, 1 out]
      n135 = property on="Channel Graph 6" class="WFGraph (strict)"(error in=w377, "YScale.NameLbl.Text"=w360) -> (error out=w376:errorcluster)  [unwired: 1 in, 1 out]
      n136 = property on="Channel Graph 7" class="WFGraph (strict)"(error in=w376, "YScale.NameLbl.Text"=w360) -> (error out=w374:errorcluster)  [unwired: 1 in, 1 out]
    }
    frame 5 {
      w383 = "NONE" ("Y Scale.Name Label.Text")
      n137 = Index Array(array=w392, index=0) -> (element=w394:string)
      n138 = property on="Channel Graph 0" class="WFGraph (strict)"(error in=w396, "YScale.NameLbl.Text"=w394) -> (error out=w403:errorcluster)  [unwired: 1 in, 1 out]
      n139 = Index Array(array=w392, index=1) -> (element=w393:string)
      n140 = property on="Channel Graph 1" class="WFGraph (strict)"(error in=w403, "YScale.NameLbl.Text"=w393) -> (error out=w402:errorcluster)  [unwired: 1 in, 1 out]
      n141 = Index Array(array=w392, index=2) -> (element=w386:string)
      n142 = property on="Channel Graph 2" class="WFGraph (strict)"(error in=w402, "YScale.NameLbl.Text"=w386) -> (error out=w401:errorcluster)  [unwired: 1 in, 1 out]
      n143 = Index Array(array=w392, index=3) -> (element=w385:string)
      n144 = property on="Channel Graph 3" class="WFGraph (strict)"(error in=w401, "YScale.NameLbl.Text"=w385) -> (error out=w400:errorcluster)  [unwired: 1 in, 1 out]
      n145 = Index Array(array=w392, index=4) -> (element=w384:string)
      n146 = property on="Channel Graph 4" class="WFGraph (strict)"(error in=w400, "YScale.NameLbl.Text"=w384) -> (error out=w399:errorcluster)  [unwired: 1 in, 1 out]
      n147 = property on="Channel Graph 5" class="WFGraph (strict)"(error in=w399, "YScale.NameLbl.Text"=w383) -> (error out=w398:errorcluster)  [unwired: 1 in, 1 out]
      n148 = property on="Channel Graph 6" class="WFGraph (strict)"(error in=w398, "YScale.NameLbl.Text"=w383) -> (error out=w397:errorcluster)  [unwired: 1 in, 1 out]
      n149 = property on="Channel Graph 7" class="WFGraph (strict)"(error in=w397, "YScale.NameLbl.Text"=w383) -> (error out=w395:errorcluster)  [unwired: 1 in, 1 out]
    }
    frame 4 {
      w404 = "NONE" ("Y Scale.Name Label.Text")
      n150 = Index Array(array=w411, index=0) -> (element=w413:string)
      n151 = property on="Channel Graph 0" class="WFGraph (strict)"(error in=w415, "YScale.NameLbl.Text"=w413) -> (error out=w422:errorcluster)  [unwired: 1 in, 1 out]
      n152 = Index Array(array=w411, index=1) -> (element=w412:string)
      n153 = property on="Channel Graph 1" class="WFGraph (strict)"(error in=w422, "YScale.NameLbl.Text"=w412) -> (error out=w421:errorcluster)  [unwired: 1 in, 1 out]
      n154 = Index Array(array=w411, index=2) -> (element=w406:string)
      n155 = property on="Channel Graph 2" class="WFGraph (strict)"(error in=w421, "YScale.NameLbl.Text"=w406) -> (error out=w420:errorcluster)  [unwired: 1 in, 1 out]
      n156 = Index Array(array=w411, index=3) -> (element=w405:string)
      n157 = property on="Channel Graph 3" class="WFGraph (strict)"(error in=w420, "YScale.NameLbl.Text"=w405) -> (error out=w419:errorcluster)  [unwired: 1 in, 1 out]
      n158 = property on="Channel Graph 4" class="WFGraph (strict)"(error in=w419, "YScale.NameLbl.Text"=w404) -> (error out=w418:errorcluster)  [unwired: 1 in, 1 out]
      n159 = property on="Channel Graph 5" class="WFGraph (strict)"(error in=w418, "YScale.NameLbl.Text"=w404) -> (error out=w417:errorcluster)  [unwired: 1 in, 1 out]
      n160 = property on="Channel Graph 6" class="WFGraph (strict)"(error in=w417, "YScale.NameLbl.Text"=w404) -> (error out=w416:errorcluster)  [unwired: 1 in, 1 out]
      n161 = property on="Channel Graph 7" class="WFGraph (strict)"(error in=w416, "YScale.NameLbl.Text"=w404) -> (error out=w414:errorcluster)  [unwired: 1 in, 1 out]
    }
    frame 3 {
      w423 = "NONE" ("Y Scale.Name Label.Text")
      n162 = Index Array(array=w428, index=0) -> (element=w430:string)
      n163 = property on="Channel Graph 0" class="WFGraph (strict)"(error in=w432, "YScale.NameLbl.Text"=w430) -> (error out=w439:errorcluster)  [unwired: 1 in, 1 out]
      n164 = Index Array(array=w428, index=1) -> (element=w429:string)
      n165 = property on="Channel Graph 1" class="WFGraph (strict)"(error in=w439, "YScale.NameLbl.Text"=w429) -> (error out=w438:errorcluster)  [unwired: 1 in, 1 out]
      n166 = Index Array(array=w428, index=2) -> (element=w424:string)
      n167 = property on="Channel Graph 2" class="WFGraph (strict)"(error in=w438, "YScale.NameLbl.Text"=w424) -> (error out=w437:errorcluster)  [unwired: 1 in, 1 out]
      n168 = property on="Channel Graph 3" class="WFGraph (strict)"(error in=w437, "YScale.NameLbl.Text"=w423) -> (error out=w436:errorcluster)  [unwired: 1 in, 1 out]
      n169 = property on="Channel Graph 4" class="WFGraph (strict)"(error in=w436, "YScale.NameLbl.Text"=w423) -> (error out=w435:errorcluster)  [unwired: 1 in, 1 out]
      n170 = property on="Channel Graph 5" class="WFGraph (strict)"(error in=w435, "YScale.NameLbl.Text"=w423) -> (error out=w434:errorcluster)  [unwired: 1 in, 1 out]
      n171 = property on="Channel Graph 6" class="WFGraph (strict)"(error in=w434, "YScale.NameLbl.Text"=w423) -> (error out=w433:errorcluster)  [unwired: 1 in, 1 out]
      n172 = property on="Channel Graph 7" class="WFGraph (strict)"(error in=w433, "YScale.NameLbl.Text"=w423) -> (error out=w431:errorcluster)  [unwired: 1 in, 1 out]
    }
    frame 2 {
      w440 = "NONE" ("Y Scale.Name Label.Text")
      n173 = Index Array(array=w443, index=0) -> (element=w445:string)
      n174 = property on="Channel Graph 0" class="WFGraph (strict)"(error in=w447, "YScale.NameLbl.Text"=w445) -> (error out=w454:errorcluster)  [unwired: 1 in, 1 out]
      n175 = Index Array(array=w443, index=1) -> (element=w444:string)
      n176 = property on="Channel Graph 1" class="WFGraph (strict)"(error in=w454, "YScale.NameLbl.Text"=w444) -> (error out=w453:errorcluster)  [unwired: 1 in, 1 out]
      n177 = property on="Channel Graph 2" class="WFGraph (strict)"(error in=w453, "YScale.NameLbl.Text"=w440) -> (error out=w452:errorcluster)  [unwired: 1 in, 1 out]
      n178 = property on="Channel Graph 3" class="WFGraph (strict)"(error in=w452, "YScale.NameLbl.Text"=w440) -> (error out=w451:errorcluster)  [unwired: 1 in, 1 out]
      n179 = property on="Channel Graph 4" class="WFGraph (strict)"(error in=w451, "YScale.NameLbl.Text"=w440) -> (error out=w450:errorcluster)  [unwired: 1 in, 1 out]
      n180 = property on="Channel Graph 5" class="WFGraph (strict)"(error in=w450, "YScale.NameLbl.Text"=w440) -> (error out=w449:errorcluster)  [unwired: 1 in, 1 out]
      n181 = property on="Channel Graph 6" class="WFGraph (strict)"(error in=w449, "YScale.NameLbl.Text"=w440) -> (error out=w448:errorcluster)  [unwired: 1 in, 1 out]
      n182 = property on="Channel Graph 7" class="WFGraph (strict)"(error in=w448, "YScale.NameLbl.Text"=w440) -> (error out=w446:errorcluster)  [unwired: 1 in, 1 out]
    }
    frame 1 {
      w455 = "NONE" ("Y Scale.Name Label.Text")
      n183 = Index Array(array=w457, index=0) -> (element=w458:string)
      n184 = property on="Channel Graph 0" class="WFGraph (strict)"(error in=w460, "YScale.NameLbl.Text"=w458) -> (error out=w467:errorcluster)  [unwired: 1 in, 1 out]
      n185 = property on="Channel Graph 1" class="WFGraph (strict)"(error in=w467, "YScale.NameLbl.Text"=w455) -> (error out=w466:errorcluster)  [unwired: 1 in, 1 out]
      n186 = property on="Channel Graph 2" class="WFGraph (strict)"(error in=w466, "YScale.NameLbl.Text"=w455) -> (error out=w465:errorcluster)  [unwired: 1 in, 1 out]
      n187 = property on="Channel Graph 3" class="WFGraph (strict)"(error in=w465, "YScale.NameLbl.Text"=w455) -> (error out=w464:errorcluster)  [unwired: 1 in, 1 out]
      n188 = property on="Channel Graph 4" class="WFGraph (strict)"(error in=w464, "YScale.NameLbl.Text"=w455) -> (error out=w463:errorcluster)  [unwired: 1 in, 1 out]
      n189 = property on="Channel Graph 5" class="WFGraph (strict)"(error in=w463, "YScale.NameLbl.Text"=w455) -> (error out=w462:errorcluster)  [unwired: 1 in, 1 out]
      n190 = property on="Channel Graph 6" class="WFGraph (strict)"(error in=w462, "YScale.NameLbl.Text"=w455) -> (error out=w461:errorcluster)  [unwired: 1 in, 1 out]
      n191 = property on="Channel Graph 7" class="WFGraph (strict)"(error in=w461, "YScale.NameLbl.Text"=w455) -> (error out=w459:errorcluster)  [unwired: 1 in, 1 out]
    }
    frame 0, Default {
      w468 = "NONE" ("Y Scale.Name Label.Text")
      n192 = property on="Channel Graph 0" class="WFGraph (strict)"(error in=w470, "YScale.NameLbl.Text"=w468) -> (error out=w477:errorcluster)  [unwired: 1 in, 1 out]
      n193 = property on="Channel Graph 1" class="WFGraph (strict)"(error in=w477, "YScale.NameLbl.Text"=w468) -> (error out=w476:errorcluster)  [unwired: 1 in, 1 out]
      n194 = property on="Channel Graph 2" class="WFGraph (strict)"(error in=w476, "YScale.NameLbl.Text"=w468) -> (error out=w475:errorcluster)  [unwired: 1 in, 1 out]
      n195 = property on="Channel Graph 3" class="WFGraph (strict)"(error in=w475, "YScale.NameLbl.Text"=w468) -> (error out=w474:errorcluster)  [unwired: 1 in, 1 out]
      n196 = property on="Channel Graph 4" class="WFGraph (strict)"(error in=w474, "YScale.NameLbl.Text"=w468) -> (error out=w473:errorcluster)  [unwired: 1 in, 1 out]
      n197 = property on="Channel Graph 5" class="WFGraph (strict)"(error in=w473, "YScale.NameLbl.Text"=w468) -> (error out=w472:errorcluster)  [unwired: 1 in, 1 out]
      n198 = property on="Channel Graph 6" class="WFGraph (strict)"(error in=w472, "YScale.NameLbl.Text"=w468) -> (error out=w471:errorcluster)  [unwired: 1 in, 1 out]
      n199 = property on="Channel Graph 7" class="WFGraph (strict)"(error in=w471, "YScale.NameLbl.Text"=w468) -> (error out=w469:errorcluster)  [unwired: 1 in, 1 out]
    }
  }
  n200 = Unbundle(w114) -> ("created path"=w40:path, w4:refnum<file>[], w43:refnum<file>[])
  n201 = for {
    tunnel: w4 -> [w480] mode=indexing
    shift-right: [w478] -> w2
    shift-left: w3 -> [w479]
    n202 = Close File(refnum=w480, error in=w479) -> (error out=w478:errorcluster)  [unwired: 1 out]
  }
  n203 = Number To Decimal String(number=w39) -> (decimal integer string=w34:string)  [unwired: 1 in]
  n204 = Get Date/Time In Seconds() -> (seconds since 1Jan1904=w84:timestamp)
  n205 = Concatenate Strings("WaveformData_", w34, ".bin" ("string")) -> (w35:string)
  n206 = Build Path(base path=w40, name or relative path=w35) -> (appended path=w32:path)
  n207 = Open/Create/Replace File(file path (use dialog)=w32, error in=w2, operation (0:open)=T8."open or create", access (0:read/write)=enum16{"read/write", "read-only", "write-only"}."read/write") -> (refnum out=w44:refnum<file>, error out=w47:errorcluster)  [unwired: 2 in, 1 out]
  n208 = call "OscilloscopeConfigurationFromCluster.vi"("error in (no error)"=w47, "output cluster"=w14) -> ("error out"=w48:errorcluster, "active channel number string array"=w30:string[], "active channel number string list"=w25:string, "IVI Refnum out"=w26:refnum<k15>)  [unwired: 6 in]
  n209 = call <instrlib>:"niDMM Initialize.vi"("error in (no error)"=w13, "Instrument Descriptor"=refnum<k15> "PXIe4081_7") -> ("error out"=w72:errorcluster, "instrument handle out"=w71:refnum<k15>)  [unwired: 8 in]
  n210 = Obtain Queue(element data type=T10 {"wfm info"=[], "wfm"=[]} ("cluster"), error in (no error)=w48) -> (queue out=w19:refnum<queue>, error out=w27:errorcluster)  [unwired: 3 in, 1 out]
  n211 = call <instrlib>:"niDMM Configure Trigger.vi"("Trigger Source"=niDMM_Trigger."Immediate", "error in (no error)"=w72, "instrument handle"=w71) -> ("error out"=w73:errorcluster, "instrument handle out"=w70:refnum<k15>)  [unwired: 7 in]
  n212 = Array Size(array=w30) -> (size(s)=w29:i32)
  n213 = Array Size(array=w30) -> (size(s)=w23:i32)
  n214 = call-poly <instrlib>:"niDMM Config Measurement.vi"("Range"=5.0, "Resolution in Digits"=w67, "error in (no error)"=w73, "Function"=niDMM_Function."DC Volts", "instrument handle"=w70) -> ("error out"=w68:errorcluster, "instrument handle out"=w69:refnum<k15>)  [unwired: 5 in]
  n215 = while {
    shift-right: [w498] -> w17
    shift-left: w26 -> [w500]
    shift-right: [w481] -> w20
    shift-left: w27 -> [w499]
    tunnel: w25 -> [w496]
    tunnel: -1 ("numSamples") -> [w495]
    tunnel: w19 -> [w493]
    tunnel: w29 -> [w490]
    shift-right: [w488] -> _
    shift-left: 0 ("x") -> [w484]
    shift-right: [w487] -> _
    shift-left: T9 {"Array"=[], "Array"=[], "Array"=[], "Array"=[], "Array"=[], "Array"=[], "Array"=[], "Array"=[]} -> [w489]
    stop <- w486 stop-if-true
    n216 = call-poly <instrlib>:"niScope Fetch (poly).vi"("timeout"=0.0, "error in"=w499, "numSamples"=w495, "channels"=w496, "instrument handle"=w500) -> ("error out"=w494:errorcluster, "wfm"=w491:i16[][], "wfm info"=w492:T19, "instrument handle out"=w498:refnum<k15>)  [unwired: 3 in]
    n217 = local read "Exiting"() -> (w486:bool)
    n218 = local read "Recording Data"() -> (w485:bool)
    n219 = case shown="True" w485 {
      tunnel: w494 -> [w776 w783]
      tunnel: w493 -> [_ w782]
      tunnel: [w776 w779] -> w482
      tunnel: w492 -> [_ w778]
      tunnel: w491 -> [_ w777]
      frame False {
      }
      frame True {
        n220 = Bundle(cluster=T10 {"wfm info"=[], "wfm"=[]}, "wfm info"=w778, "wfm"=w777) -> (w781:T10)
        n221 = Enqueue Element(queue=w782, element=w781, error in (no error)=w783) -> (error out=w779:errorcluster)  [unwired: 1 in, 2 out]
      }
    }
    n222 = case shown="True" TRUE {
      tunnel: w492 -> [_ w516]
      tunnel: w491 -> [_ w515]
      tunnel: w490 -> [_ w514]
      tunnel: w489 -> [_ w513]
      tunnel: [0 ("x") w512] -> w488
      tunnel: [T9 {"Array"=[], "Array"=[], "Array"=[], "Array"=[], "Array"=[], "Array"=[], "Array"=[], "Array"=[]} w507] -> w487
      tunnel: w484 -> [_ w510]
      tunnel: w482 -> [w501 w505]
      tunnel: [w501 w504] -> w481
      frame False {
      }
      frame True {
        n223 = Greater?(x="Reset Value", y=w510) -> (0:w509:bool)
        n224 = case shown="True" w509 {
          tunnel: w514 -> [_ w563]
          tunnel: w516 -> [_ w562]
          tunnel: w515 -> [_ w561]
          tunnel: [T9 {"Array"=[], "Array"=[], "Array"=[], "Array"=[], "Array"=[], "Array"=[], "Array"=[], "Array"=[]} w560] -> w508
          tunnel: w513 -> [_ w559]
          tunnel: [0 ("x") w558] -> w512
          tunnel: w510 -> [_ w557]
          frame False {
            n225 = disable-structure shown="Enabled" {
              frame Disabled {
                w555 = 0
                n226 = property on="Channel Graph 0" class="WFGraph (strict)"("ActYScl"=w555) -> (error out=w548:errorcluster)  [unwired: 2 in, 1 out]
                n227 = property on="Channel Graph 1" class="WFGraph (strict)"(error in=w548, "ActYScl"=w555) -> (error out=w549:errorcluster)  [unwired: 1 in, 1 out]
                n228 = property on="Channel Graph 2" class="WFGraph (strict)"(error in=w549, "ActYScl"=w555) -> (error out=w550:errorcluster)  [unwired: 1 in, 1 out]
                n229 = property on="Channel Graph 3" class="WFGraph (strict)"(error in=w550, "ActYScl"=w555) -> (error out=w551:errorcluster)  [unwired: 1 in, 1 out]
                n230 = property on="Channel Graph 4" class="WFGraph (strict)"(error in=w551, "ActYScl"=w555) -> (error out=w552:errorcluster)  [unwired: 1 in, 1 out]
                n231 = property on="Channel Graph 5" class="WFGraph (strict)"(error in=w552, "ActYScl"=w555) -> (error out=w553:errorcluster)  [unwired: 1 in, 1 out]
                n232 = property on="Channel Graph 6" class="WFGraph (strict)"(error in=w553, "ActYScl"=w555) -> (error out=w554:errorcluster)  [unwired: 1 in, 1 out]
                n233 = property on="Channel Graph 7" class="WFGraph (strict)"(error in=w554, "ActYScl"=w555) -> ()  [unwired: 1 in, 2 out]
              }
              frame Enabled {
              }
            }
          }
          frame True {
            n234 = case shown="7" w563 {
              tunnel: w562 -> [w600 w634 w665 w693 w694 w719 w759 w775]
              tunnel: w561 -> [w599 w633 w664 w692 w718 w740 w758 w774]
              tunnel: [w590 w625 w657 w686 w713 w736 w755 w772] -> w556
              tunnel: [w589 w624 w656 w685 w712 w735 w754 w771] -> w560
              tunnel: w559 -> [w588 w623 w655 w684 w711 w734 w753 w770]
              frame 8 {
                n235 = Unbundle(w588) -> ("Array"=w587:dbl[], "Array"=w586:dbl[], "Array"=w585:dbl[], "Array"=w584:dbl[], "Array"=w583:dbl[], "Array"=w582:dbl[], "Array"=w581:dbl[], "Array"=w580:dbl[])
                n236 = call "StandAloneTransient_SingleGraphCreation_DataCollection_Light.vi"("wfm"=w599, "index"=0, "wfm info"=w600) -> ("Array"=w572:dbl[])  [unwired: 8 in]
                n237 = call "StandAloneTransient_SingleGraphCreation_DataCollection_Light.vi"("wfm"=w599, "index"=1, "wfm info"=w600) -> ("Array"=w573:dbl[])  [unwired: 8 in]
                n238 = call "StandAloneTransient_SingleGraphCreation_DataCollection_Light.vi"("wfm"=w599, "index"=2, "wfm info"=w600) -> ("Array"=w574:dbl[])  [unwired: 8 in]
                n239 = call "StandAloneTransient_SingleGraphCreation_DataCollection_Light.vi"("wfm"=w599, "index"=3, "wfm info"=w600) -> ("Array"=w575:dbl[])  [unwired: 8 in]
                n240 = call "StandAloneTransient_SingleGraphCreation_DataCollection_Light.vi"("wfm"=w599, "index"=4, "wfm info"=w600) -> ("Array"=w576:dbl[])  [unwired: 8 in]
                n241 = call "StandAloneTransient_SingleGraphCreation_DataCollection_Light.vi"("wfm"=w599, "index"=5, "wfm info"=w600) -> ("Array"=w577:dbl[])  [unwired: 8 in]
                n242 = call "StandAloneTransient_SingleGraphCreation_DataCollection_Light.vi"("wfm"=w599, "index"=6, "wfm info"=w600) -> ("Array"=w578:dbl[])  [unwired: 8 in]
                n243 = call "StandAloneTransient_SingleGraphCreation_DataCollection_Light.vi"("wfm"=w599, "index"=7, "wfm info"=w600) -> ("Array"=w579:dbl[])  [unwired: 8 in]
                n244 = Insert Into Array(array=w587, new element=w572) -> (w571:dbl[])  [unwired: 1 in]
                n245 = Insert Into Array(array=w586, new element=w573) -> (w570:dbl[])  [unwired: 1 in]
                n246 = Insert Into Array(array=w585, new element=w574) -> (w569:dbl[])  [unwired: 1 in]
                n247 = Insert Into Array(array=w584, new element=w575) -> (w568:dbl[])  [unwired: 1 in]
                n248 = Insert Into Array(array=w583, new element=w576) -> (w567:dbl[])  [unwired: 1 in]
                n249 = Insert Into Array(array=w582, new element=w577) -> (w566:dbl[])  [unwired: 1 in]
                n250 = Insert Into Array(array=w581, new element=w578) -> (w565:dbl[])  [unwired: 1 in]
                n251 = Insert Into Array(array=w580, new element=w579) -> (w564:dbl[])  [unwired: 1 in]
                n252 = local write "Channel Graph 0"(w571) -> ()
                n253 = local write "Channel Graph 1"(w570) -> ()
                n254 = local write "Channel Graph 3"(w568) -> ()
                n255 = local write "Channel Graph 2"(w569) -> ()
                n256 = local write "Channel Graph 4"(w567) -> ()
                n257 = local write "Channel Graph 5"(w566) -> ()
                n258 = local write "Channel Graph 7"(w564) -> ()
                n259 = local write "Channel Graph 6"(w565) -> ()
                n260 = Build Array(w572, w573, w574, w575, w576, w577, w578, w579) -> (w590:dbl[][])
                n261 = Bundle("Array"=w571, "Array"=w570, "Array"=w569, "Array"=w568, "Array"=w567, "Array"=w566, "Array"=w565, "Array"=w564) -> (w589:T9)  [unwired: 1 in]
              }
              frame 7 {
                n262 = Unbundle(w623) -> ("Array"=w622:dbl[], "Array"=w621:dbl[], "Array"=w620:dbl[], "Array"=w619:dbl[], "Array"=w618:dbl[], "Array"=w617:dbl[], "Array"=w616:dbl[], "Array"=w601:dbl[])
                n263 = call "StandAloneTransient_SingleGraphCreation_DataCollection_Light.vi"("wfm"=w633, "index"=0, "wfm info"=w634) -> ("Array"=w609:dbl[])  [unwired: 8 in]
                n264 = call "StandAloneTransient_SingleGraphCreation_DataCollection_Light.vi"("wfm"=w633, "index"=1, "wfm info"=w634) -> ("Array"=w610:dbl[])  [unwired: 8 in]
                n265 = call "StandAloneTransient_SingleGraphCreation_DataCollection_Light.vi"("wfm"=w633, "index"=2, "wfm info"=w634) -> ("Array"=w611:dbl[])  [unwired: 8 in]
                n266 = call "StandAloneTransient_SingleGraphCreation_DataCollection_Light.vi"("wfm"=w633, "index"=3, "wfm info"=w634) -> ("Array"=w612:dbl[])  [unwired: 8 in]
                n267 = call "StandAloneTransient_SingleGraphCreation_DataCollection_Light.vi"("wfm"=w633, "index"=4, "wfm info"=w634) -> ("Array"=w613:dbl[])  [unwired: 8 in]
                n268 = call "StandAloneTransient_SingleGraphCreation_DataCollection_Light.vi"("wfm"=w633, "index"=5, "wfm info"=w634) -> ("Array"=w614:dbl[])  [unwired: 8 in]
                n269 = call "StandAloneTransient_SingleGraphCreation_DataCollection_Light.vi"("wfm"=w633, "index"=6, "wfm info"=w634) -> ("Array"=w615:dbl[])  [unwired: 8 in]
                n270 = Insert Into Array(array=w622, new element=w609) -> (w608:dbl[])  [unwired: 1 in]
                n271 = Insert Into Array(array=w621, new element=w610) -> (w607:dbl[])  [unwired: 1 in]
                n272 = Insert Into Array(array=w620, new element=w611) -> (w606:dbl[])  [unwired: 1 in]
                n273 = Insert Into Array(array=w619, new element=w612) -> (w605:dbl[])  [unwired: 1 in]
                n274 = Insert Into Array(array=w618, new element=w613) -> (w604:dbl[])  [unwired: 1 in]
                n275 = Insert Into Array(array=w617, new element=w614) -> (w603:dbl[])  [unwired: 1 in]
                n276 = Insert Into Array(array=w616, new element=w615) -> (w602:dbl[])  [unwired: 1 in]
                n277 = Build Array(w609, w610, w611, w612, w613, w614, w615) -> (w625:dbl[][])
                n278 = local write "Channel Graph 0"(w608) -> ()
                n279 = local write "Channel Graph 1"(w607) -> ()
                n280 = local write "Channel Graph 2"(w606) -> ()
                n281 = local write "Channel Graph 4"(w604) -> ()
                n282 = local write "Channel Graph 3"(w605) -> ()
                n283 = local write "Channel Graph 5"(w603) -> ()
                n284 = local write "Channel Graph 6"(w602) -> ()
                n285 = Bundle("Array"=w608, "Array"=w607, "Array"=w606, "Array"=w605, "Array"=w604, "Array"=w603, "Array"=w602, "Array"=w601) -> (w624:T9)  [unwired: 1 in]
              }
              frame 6 {
                n286 = Unbundle(w655) -> ("Array"=w654:dbl[], "Array"=w653:dbl[], "Array"=w652:dbl[], "Array"=w651:dbl[], "Array"=w650:dbl[], "Array"=w649:dbl[], "Array"=w636:dbl[], "Array"=w635:dbl[])
                n287 = call "StandAloneTransient_SingleGraphCreation_DataCollection_Light.vi"("wfm"=w664, "index"=0, "wfm info"=w665) -> ("Array"=w643:dbl[])  [unwired: 8 in]
                n288 = call "StandAloneTransient_SingleGraphCreation_DataCollection_Light.vi"("wfm"=w664, "index"=1, "wfm info"=w665) -> ("Array"=w644:dbl[])  [unwired: 8 in]
                n289 = call "StandAloneTransient_SingleGraphCreation_DataCollection_Light.vi"("wfm"=w664, "index"=2, "wfm info"=w665) -> ("Array"=w645:dbl[])  [unwired: 8 in]
                n290 = call "StandAloneTransient_SingleGraphCreation_DataCollection_Light.vi"("wfm"=w664, "index"=3, "wfm info"=w665) -> ("Array"=w646:dbl[])  [unwired: 8 in]
                n291 = call "StandAloneTransient_SingleGraphCreation_DataCollection_Light.vi"("wfm"=w664, "index"=4, "wfm info"=w665) -> ("Array"=w647:dbl[])  [unwired: 8 in]
                n292 = call "StandAloneTransient_SingleGraphCreation_DataCollection_Light.vi"("wfm"=w664, "index"=5, "wfm info"=w665) -> ("Array"=w648:dbl[])  [unwired: 8 in]
                n293 = Insert Into Array(array=w654, new element=w643) -> (w642:dbl[])  [unwired: 1 in]
                n294 = Insert Into Array(array=w653, new element=w644) -> (w641:dbl[])  [unwired: 1 in]
                n295 = Insert Into Array(array=w652, new element=w645) -> (w640:dbl[])  [unwired: 1 in]
                n296 = Insert Into Array(array=w651, new element=w646) -> (w639:dbl[])  [unwired: 1 in]
                n297 = Insert Into Array(array=w650, new element=w647) -> (w638:dbl[])  [unwired: 1 in]
                n298 = Insert Into Array(array=w649, new element=w648) -> (w637:dbl[])  [unwired: 1 in]
                n299 = Build Array(w643, w644, w645, w646, w647, w648) -> (w657:dbl[][])
                n300 = local write "Channel Graph 0"(w642) -> ()
                n301 = local write "Channel Graph 1"(w641) -> ()
                n302 = local write "Channel Graph 2"(w640) -> ()
                n303 = local write "Channel Graph 4"(w638) -> ()
                n304 = local write "Channel Graph 3"(w639) -> ()
                n305 = local write "Channel Graph 5"(w637) -> ()
                n306 = Bundle("Array"=w642, "Array"=w641, "Array"=w640, "Array"=w639, "Array"=w638, "Array"=w637, "Array"=w636, "Array"=w635) -> (w656:T9)  [unwired: 1 in]
              }
              frame 5 {
                n307 = Unbundle(w684) -> ("Array"=w683:dbl[], "Array"=w682:dbl[], "Array"=w681:dbl[], "Array"=w680:dbl[], "Array"=w679:dbl[], "Array"=w668:dbl[], "Array"=w667:dbl[], "Array"=w666:dbl[])
                n308 = call "StandAloneTransient_SingleGraphCreation_DataCollection_Light.vi"("wfm"=w692, "index"=0, "wfm info"=w693) -> ("Array"=w674:dbl[])  [unwired: 8 in]
                n309 = call "StandAloneTransient_SingleGraphCreation_DataCollection_Light.vi"("wfm"=w692, "index"=1, "wfm info"=w693) -> ("Array"=w675:dbl[])  [unwired: 8 in]
                n310 = call "StandAloneTransient_SingleGraphCreation_DataCollection_Light.vi"("wfm"=w692, "index"=2, "wfm info"=w693) -> ("Array"=w676:dbl[])  [unwired: 8 in]
                n311 = call "StandAloneTransient_SingleGraphCreation_DataCollection_Light.vi"("wfm"=w692, "index"=3, "wfm info"=w693) -> ("Array"=w677:dbl[])  [unwired: 8 in]
                n312 = call "StandAloneTransient_SingleGraphCreation_DataCollection_Light.vi"("wfm"=w692, "index"=4, "wfm info"=w693) -> ("Array"=w678:dbl[])  [unwired: 8 in]
                n313 = Insert Into Array(array=w683, new element=w674) -> (w673:dbl[])  [unwired: 1 in]
                n314 = Insert Into Array(array=w682, new element=w675) -> (w672:dbl[])  [unwired: 1 in]
                n315 = Insert Into Array(array=w681, new element=w676) -> (w671:dbl[])  [unwired: 1 in]
                n316 = Insert Into Array(array=w680, new element=w677) -> (w670:dbl[])  [unwired: 1 in]
                n317 = Insert Into Array(array=w679, new element=w678) -> (w669:dbl[])  [unwired: 1 in]
                n318 = Build Array(w674, w675, w676, w677, w678) -> (w686:dbl[][])
                n319 = local write "Channel Graph 0"(w673) -> ()
                n320 = local write "Channel Graph 1"(w672) -> ()
                n321 = local write "Channel Graph 2"(w671) -> ()
                n322 = local write "Channel Graph 4"(w669) -> ()
                n323 = local write "Channel Graph 3"(w670) -> ()
                n324 = Bundle("Array"=w673, "Array"=w672, "Array"=w671, "Array"=w670, "Array"=w669, "Array"=w668, "Array"=w667, "Array"=w666) -> (w685:T9)  [unwired: 1 in]
              }
              frame 4 {
                n325 = Unbundle(w711) -> ("Array"=w710:dbl[], "Array"=w709:dbl[], "Array"=w708:dbl[], "Array"=w707:dbl[], "Array"=w698:dbl[], "Array"=w697:dbl[], "Array"=w696:dbl[], "Array"=w695:dbl[])
                n326 = call "StandAloneTransient_SingleGraphCreation_DataCollection_Light.vi"("wfm"=w718, "index"=0, "wfm info"=w694) -> ("Array"=w703:dbl[])  [unwired: 8 in]
                n327 = call "StandAloneTransient_SingleGraphCreation_DataCollection_Light.vi"("wfm"=w718, "index"=1, "wfm info"=w694) -> ("Array"=w704:dbl[])  [unwired: 8 in]
                n328 = call "StandAloneTransient_SingleGraphCreation_DataCollection_Light.vi"("wfm"=w718, "index"=2, "wfm info"=w694) -> ("Array"=w705:dbl[])  [unwired: 8 in]
                n329 = call "StandAloneTransient_SingleGraphCreation_DataCollection_Light.vi"("wfm"=w718, "index"=3, "wfm info"=w694) -> ("Array"=w706:dbl[])  [unwired: 8 in]
                n330 = Insert Into Array(array=w710, new element=w703) -> (w702:dbl[])  [unwired: 1 in]
                n331 = Insert Into Array(array=w709, new element=w704) -> (w701:dbl[])  [unwired: 1 in]
                n332 = Insert Into Array(array=w708, new element=w705) -> (w700:dbl[])  [unwired: 1 in]
                n333 = Insert Into Array(array=w707, new element=w706) -> (w699:dbl[])  [unwired: 1 in]
                n334 = Build Array(w703, w704, w705, w706) -> (w713:dbl[][])
                n335 = local write "Channel Graph 0"(w702) -> ()
                n336 = local write "Channel Graph 1"(w701) -> ()
                n337 = local write "Channel Graph 2"(w700) -> ()
                n338 = local write "Channel Graph 3"(w699) -> ()
                n339 = Bundle("Array"=w702, "Array"=w701, "Array"=w700, "Array"=w699, "Array"=w698, "Array"=w697, "Array"=w696, "Array"=w695) -> (w712:T9)  [unwired: 1 in]
              }
              frame 3 {
                n340 = Unbundle(w734) -> ("Array"=w733:dbl[], "Array"=w732:dbl[], "Array"=w731:dbl[], "Array"=w724:dbl[], "Array"=w723:dbl[], "Array"=w722:dbl[], "Array"=w721:dbl[], "Array"=w720:dbl[])
                n341 = call "StandAloneTransient_SingleGraphCreation_DataCollection_Light.vi"("wfm"=w740, "index"=0, "wfm info"=w719) -> ("Array"=w728:dbl[])  [unwired: 8 in]
                n342 = call "StandAloneTransient_SingleGraphCreation_DataCollection_Light.vi"("wfm"=w740, "index"=1, "wfm info"=w719) -> ("Array"=w729:dbl[])  [unwired: 8 in]
                n343 = call "StandAloneTransient_SingleGraphCreation_DataCollection_Light.vi"("wfm"=w740, "index"=2, "wfm info"=w719) -> ("Array"=w730:dbl[])  [unwired: 8 in]
                n344 = Insert Into Array(array=w733, new element=w728) -> (w727:dbl[])  [unwired: 1 in]
                n345 = Insert Into Array(array=w732, new element=w729) -> (w726:dbl[])  [unwired: 1 in]
                n346 = Insert Into Array(array=w731, new element=w730) -> (w725:dbl[])  [unwired: 1 in]
                n347 = local write "Channel Graph 0"(w727) -> ()
                n348 = local write "Channel Graph 1"(w726) -> ()
                n349 = local write "Channel Graph 2"(w725) -> ()
                n350 = Build Array(w728, w729, w730) -> (w736:dbl[][])
                n351 = Bundle("Array"=w727, "Array"=w726, "Array"=w725, "Array"=w724, "Array"=w723, "Array"=w722, "Array"=w721, "Array"=w720) -> (w735:T9)  [unwired: 1 in]
              }
              frame 2 {
                n352 = Unbundle(w753) -> ("Array"=w752:dbl[], "Array"=w751:dbl[], "Array"=w746:dbl[], "Array"=w745:dbl[], "Array"=w744:dbl[], "Array"=w743:dbl[], "Array"=w742:dbl[], "Array"=w741:dbl[])
                n353 = call "StandAloneTransient_SingleGraphCreation_DataCollection_Light.vi"("wfm"=w758, "index"=0, "wfm info"=w759) -> ("Array"=w749:dbl[])  [unwired: 8 in]
                n354 = call "StandAloneTransient_SingleGraphCreation_DataCollection_Light.vi"("wfm"=w758, "index"=1, "wfm info"=w759) -> ("Array"=w750:dbl[])  [unwired: 8 in]
                n355 = Insert Into Array(array=w752, new element=w749) -> (w748:dbl[])  [unwired: 1 in]
                n356 = Insert Into Array(array=w751, new element=w750) -> (w747:dbl[])  [unwired: 1 in]
                n357 = Build Array(w749, w750) -> (w755:dbl[][])
                n358 = local write "Channel Graph 0"(w748) -> ()
                n359 = local write "Channel Graph 1"(w747) -> ()
                n360 = Bundle("Array"=w748, "Array"=w747, "Array"=w746, "Array"=w745, "Array"=w744, "Array"=w743, "Array"=w742, "Array"=w741) -> (w754:T9)  [unwired: 1 in]
              }
              frame 1, Default {
                n361 = Unbundle(w770) -> ("Array"=w769:dbl[], "Array"=w766:dbl[], "Array"=w765:dbl[], "Array"=w764:dbl[], "Array"=w763:dbl[], "Array"=w762:dbl[], "Array"=w761:dbl[], "Array"=w760:dbl[])
                n362 = call "StandAloneTransient_SingleGraphCreation_DataCollection_Light.vi"("wfm"=w774, "index"=0, "wfm info"=w775) -> ("Array"=w768:dbl[])  [unwired: 8 in]
                n363 = Insert Into Array(array=w769, new element=w768) -> (w767:dbl[])  [unwired: 1 in]
                n364 = Build Array(w768) -> (w772:dbl[][])
                n365 = local write "Channel Graph 0"(w767) -> ()
                n366 = Bundle("Array"=w767, "Array"=w766, "Array"=w765, "Array"=w764, "Array"=w763, "Array"=w762, "Array"=w761, "Array"=w760) -> (w771:T9)  [unwired: 1 in]
              }
            }
            "Pryor's Graph" <- w556
            n367 = Increment(x=w557) -> (x+1=w558:i32)
          }
        }
        n368 = case shown="True" "Oscope Range Update" {
          tunnel: w508 -> [w518 w545]
          tunnel: [w518 w545] -> w507
          tunnel: w505 -> [w517 w519]
          tunnel: [w517 w520] -> w504
          frame False {
          }
          frame True {
            w537 = 0
            n369 = property on="Channel Graph 0" class="WFGraph (strict)"(error in=w519, "YScale.ScaleFit"=w537, "YScale.Maximum"="Max Range 0", "YScale.Minimum"="Min Range 0") -> (error out=w544:errorcluster)  [unwired: 1 in, 1 out]
            n370 = property on="Channel Graph 1" class="WFGraph (strict)"(error in=w544, "YScale.ScaleFit"=w537, "YScale.Maximum"="Max Range 1", "YScale.Minimum"="Min Range 1") -> (error out=w543:errorcluster)  [unwired: 1 in, 1 out]
            n371 = property on="Channel Graph 2" class="WFGraph (strict)"(error in=w543, "YScale.ScaleFit"=w537, "YScale.Maximum"="Max Range 2", "YScale.Minimum"="Min Range 2") -> (error out=w542:errorcluster)  [unwired: 1 in, 1 out]
            n372 = property on="Channel Graph 3" class="WFGraph (strict)"(error in=w542, "YScale.ScaleFit"=w537, "YScale.Maximum"="Max Range 3", "YScale.Minimum"="Min Range 3") -> (error out=w541:errorcluster)  [unwired: 1 in, 1 out]
            n373 = property on="Channel Graph 4" class="WFGraph (strict)"(error in=w541, "YScale.ScaleFit"=w537, "YScale.Maximum"="Max Range 4", "YScale.Minimum"="Min Range 4") -> (error out=w540:errorcluster)  [unwired: 1 in, 1 out]
            n374 = property on="Channel Graph 5" class="WFGraph (strict)"(error in=w540, "YScale.ScaleFit"=w537, "YScale.Maximum"="Max Range 5", "YScale.Minimum"="Min Range 5") -> (error out=w539:errorcluster)  [unwired: 1 in, 1 out]
            n375 = property on="Channel Graph 6" class="WFGraph (strict)"(error in=w539, "YScale.ScaleFit"=w537, "YScale.Maximum"="Max Range 6", "YScale.Minimum"="Min Range 6") -> (error out=w538:errorcluster)  [unwired: 1 in, 1 out]
            n376 = property on="Channel Graph 7" class="WFGraph (strict)"(error in=w538, "YScale.ScaleFit"=w537, "YScale.Maximum"="Max Range 7", "YScale.Minimum"="Min Range 7") -> (error out=w520:errorcluster)  [unwired: 1 in, 1 out]
          }
        }
      }
    }
  }
  n377 = while {
    shift-right: [w805] -> w42
    shift-left: w27 -> [w808]
    tunnel: w19 -> [w807]
    shift-right: [w803] -> _
    shift-left: 0 ("x") -> [w804]
    tunnel: w23 -> [w802]
    shift-right: [w801] -> _
    shift-left: T9 {"Array"=[], "Array"=[], "Array"=[], "Array"=[], "Array"=[], "Array"=[], "Array"=[], "Array"=[]} -> [w800]
    shift-right: [w789] -> _
    shift-left: w39 -> [w790]
    tunnel: w40 -> [w788]
    shift-right: [w787] -> w45
    shift-left: w44 -> [w786]
    shift-right: [w784] -> _
    shift-left: 0 ("y") -> [w785]
    stop <- w792 stop-if-true
    n378 = Get Queue Status(queue=w807, error in (no error)=w808) -> (queue out=w810:refnum<queue>, error out=w811:errorcluster, # elements in queue=w791:i32)  [unwired: 1 in, 5 out]
    n379 = Dequeue Element(queue=w810, timeout in ms (-1)=100, error in (no error)=w811) -> (element=w798:T10, error out=w806:errorcluster)  [unwired: 2 out]
    n380 = Unbundle By Name(w798) -> ("wfm info"=w797:T19, "wfm"=w799:i16[][])
    n381 = Array Size(array=w797) -> (size(s)=w796:i32)
    n382 = Greater Than 0?(x=w796) -> (x > 0?=w795:bool)
    n383 = disable-structure shown="Enabled" {
      disable-tunnel: w806 -> [w822 w1079 w1111]
      disable-tunnel: [w821 w1072 w1107] -> w805
      disable-tunnel: w804 -> [w819 w1080 w1112]
      disable-tunnel: [w818 w1080 w1112] -> w803
      disable-tunnel: w802 -> [w817 _ _]
      disable-tunnel: [w816 w1081 w1113] -> w801
      disable-tunnel: w800 -> [w815 w1081 w1113]
      disable-tunnel: w799 -> [w814 w1077 w1109]
      disable-tunnel: w797 -> [w813 w1078 w1110]
      disable-tunnel: w795 -> [w812 w1076 w1108]
      disable-tunnel: w790 -> [_ _ w1103]
      disable-tunnel: [_ 0 w1105] -> w789
      disable-tunnel: w786 -> [_ w1075 w1100]
      disable-tunnel: w788 -> [_ _ w1101]
      disable-tunnel: [_ w1071 w1098] -> w787
      disable-tunnel: w785 -> [_ _ w1097]
      disable-tunnel: [_ 0 w1096] -> w784
      frame Disabled {
        n384 = case shown="True" w812 {
          tunnel: w822 -> [w825 w838]
          tunnel: [w825 w837] -> w821
          tunnel: "Reset Value 2" -> [_ w836]
          tunnel: w819 -> [w824 w835]
          tunnel: [w824 w834] -> w818
          tunnel: w817 -> [_ w832]
          tunnel: [w823 w831] -> w816
          tunnel: w815 -> [w823 w830]
          tunnel: w813 -> [_ w827]
          tunnel: w814 -> [_ w826]
          frame False {
          }
          frame True {
            n385 = Greater?(x=w836, y=w835) -> (0:w828:bool)
            n386 = And(y=w828) -> (x=w833:bool, x .and. y?=w829:bool)
            n387 = case shown="True" w829 {
              tunnel: w832 -> [_ w850]
              tunnel: w827 -> [_ w849]
              tunnel: w826 -> [_ w848]
              tunnel: w838 -> [w839 w847]
              tunnel: [T9 {"Array"=[], "Array"=[], "Array"=[], "Array"=[], "Array"=[], "Array"=[], "Array"=[], "Array"=[]} w846] -> w831
              tunnel: w830 -> [_ w845]
              tunnel: [w839 w844] -> w837
              tunnel: [0 ("x") w843] -> w834
              tunnel: w835 -> [_ w842]
              frame False {
              }
              frame True {
                n388 = case shown="8" w850 {
                  tunnel: w849 -> [w888 w923 w955 w984 w985 w1011 w1053 w1070]
                  tunnel: w848 -> [w887 w922 w954 w983 w1010 w1033 w1052 w1069]
                  tunnel: [w878 w914 w947 w977 w1005 w1029 w1049 w1067] -> _
                  tunnel: [w877 w913 w946 w976 w1004 w1028 w1048 w1066] -> w844
                  tunnel: w847 -> [w877 w913 w946 w976 w1004 w1028 w1048 w1066]
                  tunnel: [w876 w912 w945 w975 w1003 w1027 w1047 w1065] -> w846
                  tunnel: w845 -> [w875 w911 w944 w974 w1002 w1026 w1046 w1064]
                  frame 8 {
                    n389 = Unbundle(w875) -> ("Array"=w874:dbl[], "Array"=w873:dbl[], "Array"=w872:dbl[], "Array"=w871:dbl[], "Array"=w870:dbl[], "Array"=w869:dbl[], "Array"=w868:dbl[], "Array"=w867:dbl[])
                    n390 = call "StandAloneTransient_SingleGraphCreation_DataCollection_Light.vi"("wfm"=w887, "index"=0, "wfm info"=w888) -> ("Array"=w859:dbl[])  [unwired: 8 in]
                    n391 = call "StandAloneTransient_SingleGraphCreation_DataCollection_Light.vi"("wfm"=w887, "index"=1, "wfm info"=w888) -> ("Array"=w860:dbl[])  [unwired: 8 in]
                    n392 = call "StandAloneTransient_SingleGraphCreation_DataCollection_Light.vi"("wfm"=w887, "index"=2, "wfm info"=w888) -> ("Array"=w861:dbl[])  [unwired: 8 in]
                    n393 = call "StandAloneTransient_SingleGraphCreation_DataCollection_Light.vi"("wfm"=w887, "index"=3, "wfm info"=w888) -> ("Array"=w862:dbl[])  [unwired: 8 in]
                    n394 = call "StandAloneTransient_SingleGraphCreation_DataCollection_Light.vi"("wfm"=w887, "index"=4, "wfm info"=w888) -> ("Array"=w863:dbl[])  [unwired: 8 in]
                    n395 = call "StandAloneTransient_SingleGraphCreation_DataCollection_Light.vi"("wfm"=w887, "index"=5, "wfm info"=w888) -> ("Array"=w864:dbl[])  [unwired: 8 in]
                    n396 = call "StandAloneTransient_SingleGraphCreation_DataCollection_Light.vi"("wfm"=w887, "index"=6, "wfm info"=w888) -> ("Array"=w865:dbl[])  [unwired: 8 in]
                    n397 = call "StandAloneTransient_SingleGraphCreation_DataCollection_Light.vi"("wfm"=w887, "index"=7, "wfm info"=w888) -> ("Array"=w866:dbl[])  [unwired: 8 in]
                    n398 = Insert Into Array(array=w874, new element=w859) -> (w858:dbl[])  [unwired: 1 in]
                    n399 = Insert Into Array(array=w873, new element=w860) -> (w857:dbl[])  [unwired: 1 in]
                    n400 = Insert Into Array(array=w872, new element=w861) -> (w856:dbl[])  [unwired: 1 in]
                    n401 = Insert Into Array(array=w871, new element=w862) -> (w855:dbl[])  [unwired: 1 in]
                    n402 = Insert Into Array(array=w870, new element=w863) -> (w854:dbl[])  [unwired: 1 in]
                    n403 = Insert Into Array(array=w869, new element=w864) -> (w853:dbl[])  [unwired: 1 in]
                    n404 = Insert Into Array(array=w868, new element=w865) -> (w852:dbl[])  [unwired: 1 in]
                    n405 = Insert Into Array(array=w867, new element=w866) -> (w851:dbl[])  [unwired: 1 in]
                    n406 = Build Array(w859, w860, w861, w862, w863, w864, w865, w866) -> (w878:dbl[][])
                    n407 = local write item#-1(w858) -> ()
                    n408 = local write item#-1(w857) -> ()
                    n409 = local write item#-1(w855) -> ()
                    n410 = local write item#-1(w856) -> ()
                    n411 = local write item#-1(w854) -> ()
                    n412 = local write item#-1(w853) -> ()
                    n413 = local write item#-1(w851) -> ()
                    n414 = local write item#-1(w852) -> ()
                    n415 = Bundle("Array"=w858, "Array"=w857, "Array"=w856, "Array"=w855, "Array"=w854, "Array"=w853, "Array"=w852, "Array"=w851) -> (w876:T9)  [unwired: 1 in]
                  }
                  frame 7 {
                    n416 = Unbundle(w911) -> ("Array"=w910:dbl[], "Array"=w909:dbl[], "Array"=w908:dbl[], "Array"=w907:dbl[], "Array"=w906:dbl[], "Array"=w905:dbl[], "Array"=w904:dbl[], "Array"=w889:dbl[])
                    n417 = call "StandAloneTransient_SingleGraphCreation_DataCollection_Light.vi"("wfm"=w922, "index"=0, "wfm info"=w923) -> ("Array"=w897:dbl[])  [unwired: 8 in]
                    n418 = call "StandAloneTransient_SingleGraphCreation_DataCollection_Light.vi"("wfm"=w922, "index"=1, "wfm info"=w923) -> ("Array"=w898:dbl[])  [unwired: 8 in]
                    n419 = call "StandAloneTransient_SingleGraphCreation_DataCollection_Light.vi"("wfm"=w922, "index"=2, "wfm info"=w923) -> ("Array"=w899:dbl[])  [unwired: 8 in]
                    n420 = call "StandAloneTransient_SingleGraphCreation_DataCollection_Light.vi"("wfm"=w922, "index"=3, "wfm info"=w923) -> ("Array"=w900:dbl[])  [unwired: 8 in]
                    n421 = call "StandAloneTransient_SingleGraphCreation_DataCollection_Light.vi"("wfm"=w922, "index"=4, "wfm info"=w923) -> ("Array"=w901:dbl[])  [unwired: 8 in]
                    n422 = call "StandAloneTransient_SingleGraphCreation_DataCollection_Light.vi"("wfm"=w922, "index"=5, "wfm info"=w923) -> ("Array"=w902:dbl[])  [unwired: 8 in]
                    n423 = call "StandAloneTransient_SingleGraphCreation_DataCollection_Light.vi"("wfm"=w922, "index"=6, "wfm info"=w923) -> ("Array"=w903:dbl[])  [unwired: 8 in]
                    n424 = Insert Into Array(array=w910, new element=w897) -> (w896:dbl[])  [unwired: 1 in]
                    n425 = Insert Into Array(array=w909, new element=w898) -> (w895:dbl[])  [unwired: 1 in]
                    n426 = Insert Into Array(array=w908, new element=w899) -> (w894:dbl[])  [unwired: 1 in]
                    n427 = Insert Into Array(array=w907, new element=w900) -> (w893:dbl[])  [unwired: 1 in]
                    n428 = Insert Into Array(array=w906, new element=w901) -> (w892:dbl[])  [unwired: 1 in]
                    n429 = Insert Into Array(array=w905, new element=w902) -> (w891:dbl[])  [unwired: 1 in]
                    n430 = Insert Into Array(array=w904, new element=w903) -> (w890:dbl[])  [unwired: 1 in]
                    n431 = Build Array(w897, w898, w899, w900, w901, w902, w903) -> (w914:dbl[][])
                    n432 = local write item#-1(w896) -> ()
                    n433 = local write item#-1(w895) -> ()
                    n434 = local write item#-1(w894) -> ()
                    n435 = local write item#-1(w892) -> ()
                    n436 = local write item#-1(w893) -> ()
                    n437 = local write item#-1(w891) -> ()
                    n438 = local write item#-1(w890) -> ()
                    n439 = Bundle("Array"=w896, "Array"=w895, "Array"=w894, "Array"=w893, "Array"=w892, "Array"=w891, "Array"=w890, "Array"=w889) -> (w912:T9)  [unwired: 1 in]
                  }
                  frame 6 {
                    n440 = Unbundle(w944) -> ("Array"=w943:dbl[], "Array"=w942:dbl[], "Array"=w941:dbl[], "Array"=w940:dbl[], "Array"=w939:dbl[], "Array"=w938:dbl[], "Array"=w925:dbl[], "Array"=w924:dbl[])
                    n441 = call "StandAloneTransient_SingleGraphCreation_DataCollection_Light.vi"("wfm"=w954, "index"=0, "wfm info"=w955) -> ("Array"=w932:dbl[])  [unwired: 8 in]
                    n442 = call "StandAloneTransient_SingleGraphCreation_DataCollection_Light.vi"("wfm"=w954, "index"=1, "wfm info"=w955) -> ("Array"=w933:dbl[])  [unwired: 8 in]
                    n443 = call "StandAloneTransient_SingleGraphCreation_DataCollection_Light.vi"("wfm"=w954, "index"=2, "wfm info"=w955) -> ("Array"=w934:dbl[])  [unwired: 8 in]
                    n444 = call "StandAloneTransient_SingleGraphCreation_DataCollection_Light.vi"("wfm"=w954, "index"=3, "wfm info"=w955) -> ("Array"=w935:dbl[])  [unwired: 8 in]
                    n445 = call "StandAloneTransient_SingleGraphCreation_DataCollection_Light.vi"("wfm"=w954, "index"=4, "wfm info"=w955) -> ("Array"=w936:dbl[])  [unwired: 8 in]
                    n446 = call "StandAloneTransient_SingleGraphCreation_DataCollection_Light.vi"("wfm"=w954, "index"=5, "wfm info"=w955) -> ("Array"=w937:dbl[])  [unwired: 8 in]
                    n447 = Insert Into Array(array=w943, new element=w932) -> (w931:dbl[])  [unwired: 1 in]
                    n448 = Insert Into Array(array=w942, new element=w933) -> (w930:dbl[])  [unwired: 1 in]
                    n449 = Insert Into Array(array=w941, new element=w934) -> (w929:dbl[])  [unwired: 1 in]
                    n450 = Insert Into Array(array=w940, new element=w935) -> (w928:dbl[])  [unwired: 1 in]
                    n451 = Insert Into Array(array=w939, new element=w936) -> (w927:dbl[])  [unwired: 1 in]
                    n452 = Insert Into Array(array=w938, new element=w937) -> (w926:dbl[])  [unwired: 1 in]
                    n453 = Build Array(w932, w933, w934, w935, w936, w937) -> (w947:dbl[][])
                    n454 = local write item#-1(w931) -> ()
                    n455 = local write item#-1(w930) -> ()
                    n456 = local write item#-1(w929) -> ()
                    n457 = local write item#-1(w927) -> ()
                    n458 = local write item#-1(w928) -> ()
                    n459 = local write item#-1(w926) -> ()
                    n460 = Bundle("Array"=w931, "Array"=w930, "Array"=w929, "Array"=w928, "Array"=w927, "Array"=w926, "Array"=w925, "Array"=w924) -> (w945:T9)  [unwired: 1 in]
                  }
                  frame 5 {
                    n461 = Unbundle(w974) -> ("Array"=w973:dbl[], "Array"=w972:dbl[], "Array"=w971:dbl[], "Array"=w970:dbl[], "Array"=w969:dbl[], "Array"=w958:dbl[], "Array"=w957:dbl[], "Array"=w956:dbl[])
                    n462 = call "StandAloneTransient_SingleGraphCreation_DataCollection_Light.vi"("wfm"=w983, "index"=0, "wfm info"=w984) -> ("Array"=w964:dbl[])  [unwired: 8 in]
                    n463 = call "StandAloneTransient_SingleGraphCreation_DataCollection_Light.vi"("wfm"=w983, "index"=1, "wfm info"=w984) -> ("Array"=w965:dbl[])  [unwired: 8 in]
                    n464 = call "StandAloneTransient_SingleGraphCreation_DataCollection_Light.vi"("wfm"=w983, "index"=2, "wfm info"=w984) -> ("Array"=w966:dbl[])  [unwired: 8 in]
                    n465 = call "StandAloneTransient_SingleGraphCreation_DataCollection_Light.vi"("wfm"=w983, "index"=3, "wfm info"=w984) -> ("Array"=w967:dbl[])  [unwired: 8 in]
                    n466 = call "StandAloneTransient_SingleGraphCreation_DataCollection_Light.vi"("wfm"=w983, "index"=4, "wfm info"=w984) -> ("Array"=w968:dbl[])  [unwired: 8 in]
                    n467 = Insert Into Array(array=w973, new element=w964) -> (w963:dbl[])  [unwired: 1 in]
                    n468 = Insert Into Array(array=w972, new element=w965) -> (w962:dbl[])  [unwired: 1 in]
                    n469 = Insert Into Array(array=w971, new element=w966) -> (w961:dbl[])  [unwired: 1 in]
                    n470 = Insert Into Array(array=w970, new element=w967) -> (w960:dbl[])  [unwired: 1 in]
                    n471 = Insert Into Array(array=w969, new element=w968) -> (w959:dbl[])  [unwired: 1 in]
                    n472 = Build Array(w964, w965, w966, w967, w968) -> (w977:dbl[][])
                    n473 = local write item#-1(w963) -> ()
                    n474 = local write item#-1(w962) -> ()
                    n475 = local write item#-1(w961) -> ()
                    n476 = local write item#-1(w959) -> ()
                    n477 = local write item#-1(w960) -> ()
                    n478 = Bundle("Array"=w963, "Array"=w962, "Array"=w961, "Array"=w960, "Array"=w959, "Array"=w958, "Array"=w957, "Array"=w956) -> (w975:T9)  [unwired: 1 in]
                  }
                  frame 4 {
                    n479 = Unbundle(w1002) -> ("Array"=w1001:dbl[], "Array"=w1000:dbl[], "Array"=w999:dbl[], "Array"=w998:dbl[], "Array"=w989:dbl[], "Array"=w988:dbl[], "Array"=w987:dbl[], "Array"=w986:dbl[])
                    n480 = call "StandAloneTransient_SingleGraphCreation_DataCollection_Light.vi"("wfm"=w1010, "index"=0, "wfm info"=w985) -> ("Array"=w994:dbl[])  [unwired: 8 in]
                    n481 = call "StandAloneTransient_SingleGraphCreation_DataCollection_Light.vi"("wfm"=w1010, "index"=1, "wfm info"=w985) -> ("Array"=w995:dbl[])  [unwired: 8 in]
                    n482 = call "StandAloneTransient_SingleGraphCreation_DataCollection_Light.vi"("wfm"=w1010, "index"=2, "wfm info"=w985) -> ("Array"=w996:dbl[])  [unwired: 8 in]
                    n483 = call "StandAloneTransient_SingleGraphCreation_DataCollection_Light.vi"("wfm"=w1010, "index"=3, "wfm info"=w985) -> ("Array"=w997:dbl[])  [unwired: 8 in]
                    n484 = Insert Into Array(array=w1001, new element=w994) -> (w993:dbl[])  [unwired: 1 in]
                    n485 = Insert Into Array(array=w1000, new element=w995) -> (w992:dbl[])  [unwired: 1 in]
                    n486 = Insert Into Array(array=w999, new element=w996) -> (w991:dbl[])  [unwired: 1 in]
                    n487 = Insert Into Array(array=w998, new element=w997) -> (w990:dbl[])  [unwired: 1 in]
                    n488 = Build Array(w994, w995, w996, w997) -> (w1005:dbl[][])
                    n489 = local write item#-1(w993) -> ()
                    n490 = local write item#-1(w992) -> ()
                    n491 = local write item#-1(w991) -> ()
                    n492 = local write item#-1(w990) -> ()
                    n493 = Bundle("Array"=w993, "Array"=w992, "Array"=w991, "Array"=w990, "Array"=w989, "Array"=w988, "Array"=w987, "Array"=w986) -> (w1003:T9)  [unwired: 1 in]
                  }
                  frame 3 {
                    n494 = Unbundle(w1026) -> ("Array"=w1025:dbl[], "Array"=w1024:dbl[], "Array"=w1023:dbl[], "Array"=w1016:dbl[], "Array"=w1015:dbl[], "Array"=w1014:dbl[], "Array"=w1013:dbl[], "Array"=w1012:dbl[])
                    n495 = call "StandAloneTransient_SingleGraphCreation_DataCollection_Light.vi"("wfm"=w1033, "index"=0, "wfm info"=w1011) -> ("Array"=w1020:dbl[])  [unwired: 8 in]
                    n496 = call "StandAloneTransient_SingleGraphCreation_DataCollection_Light.vi"("wfm"=w1033, "index"=1, "wfm info"=w1011) -> ("Array"=w1021:dbl[])  [unwired: 8 in]
                    n497 = call "StandAloneTransient_SingleGraphCreation_DataCollection_Light.vi"("wfm"=w1033, "index"=2, "wfm info"=w1011) -> ("Array"=w1022:dbl[])  [unwired: 8 in]
                    n498 = Insert Into Array(array=w1025, new element=w1020) -> (w1019:dbl[])  [unwired: 1 in]
                    n499 = Insert Into Array(array=w1024, new element=w1021) -> (w1018:dbl[])  [unwired: 1 in]
                    n500 = Insert Into Array(array=w1023, new element=w1022) -> (w1017:dbl[])  [unwired: 1 in]
                    n501 = local write item#-1(w1019) -> ()
                    n502 = local write item#-1(w1018) -> ()
                    n503 = local write item#-1(w1017) -> ()
                    n504 = Build Array(w1020, w1021, w1022) -> (w1029:dbl[][])
                    n505 = Bundle("Array"=w1019, "Array"=w1018, "Array"=w1017, "Array"=w1016, "Array"=w1015, "Array"=w1014, "Array"=w1013, "Array"=w1012) -> (w1027:T9)  [unwired: 1 in]
                  }
                  frame 2 {
                    n506 = Unbundle(w1046) -> ("Array"=w1045:dbl[], "Array"=w1044:dbl[], "Array"=w1039:dbl[], "Array"=w1038:dbl[], "Array"=w1037:dbl[], "Array"=w1036:dbl[], "Array"=w1035:dbl[], "Array"=w1034:dbl[])
                    n507 = call "StandAloneTransient_SingleGraphCreation_DataCollection_Light.vi"("wfm"=w1052, "index"=0, "wfm info"=w1053) -> ("Array"=w1042:dbl[])  [unwired: 8 in]
                    n508 = call "StandAloneTransient_SingleGraphCreation_DataCollection_Light.vi"("wfm"=w1052, "index"=1, "wfm info"=w1053) -> ("Array"=w1043:dbl[])  [unwired: 8 in]
                    n509 = Insert Into Array(array=w1045, new element=w1042) -> (w1041:dbl[])  [unwired: 1 in]
                    n510 = Insert Into Array(array=w1044, new element=w1043) -> (w1040:dbl[])  [unwired: 1 in]
                    n511 = Build Array(w1042, w1043) -> (w1049:dbl[][])
                    n512 = local write item#-1(w1041) -> ()
                    n513 = local write item#-1(w1040) -> ()
                    n514 = Bundle("Array"=w1041, "Array"=w1040, "Array"=w1039, "Array"=w1038, "Array"=w1037, "Array"=w1036, "Array"=w1035, "Array"=w1034) -> (w1047:T9)  [unwired: 1 in]
                  }
                  frame 1, Default {
                    n515 = Unbundle(w1064) -> ("Array"=w1063:dbl[], "Array"=w1060:dbl[], "Array"=w1059:dbl[], "Array"=w1058:dbl[], "Array"=w1057:dbl[], "Array"=w1056:dbl[], "Array"=w1055:dbl[], "Array"=w1054:dbl[])
                    n516 = call "StandAloneTransient_SingleGraphCreation_DataCollection_Light.vi"("wfm"=w1069, "index"=0, "wfm info"=w1070) -> ("Array"=w1062:dbl[])  [unwired: 8 in]
                    n517 = Insert Into Array(array=w1063, new element=w1062) -> (w1061:dbl[])  [unwired: 1 in]
                    n518 = Build Array(w1062) -> (w1067:dbl[][])
                    n519 = local write item#-1(w1061) -> ()
                    n520 = Bundle("Array"=w1061, "Array"=w1060, "Array"=w1059, "Array"=w1058, "Array"=w1057, "Array"=w1056, "Array"=w1055, "Array"=w1054) -> (w1065:T9)  [unwired: 1 in]
                  }
                }
                n521 = Increment(x=w842) -> (x+1=w843:i32)
              }
            }
          }
        }
      }
      frame Enabled {
        # "single file"
        n522 = case shown="True" w1076 {
          tunnel: w1079 -> [w1083 w1090]
          tunnel: [w1083 w1089] -> w1072
          tunnel: w1078 -> [_ w1087]
          tunnel: w1077 -> [_ w1086]
          tunnel: w1075 -> [w1082 w1085]
          tunnel: [w1082 w1084] -> w1071
          frame False {
          }
          frame True {
            n523 = Bundle("wfm info"=w1087, "wfm"=w1086) -> (w1088:T10)  [unwired: 1 in]
            n524 = Set File Position(refnum=w1085, from (0:start)=enum16{"start", "end", "current"}."current", error in=w1090) -> (refnum out=w1094:refnum<file>, error out=w1095:errorcluster)  [unwired: 1 in]
            n525 = Write to Binary File(file (use dialog)=w1094, data=w1088, error in=w1095, 5:FALSE ("prepend array or string size? (T)"), 9:T20."little-endian" ("byte order (0:big-endian, network order)")) -> (refnum out=w1084:refnum<file>, error out=w1089:errorcluster)  [unwired: 1 in, 1 out]
          }
        }
      }
      frame Disabled {
        # "Breaking up the data into multiple files."
        n526 = case shown="True" w1108 {
          tunnel: w1111 -> [w1149 w1156]
          tunnel: [w1149 w1155] -> w1106
          tunnel: w1110 -> [_ w1153]
          tunnel: w1109 -> [_ w1152]
          tunnel: w1100 -> [w1148 w1151]
          tunnel: [w1148 w1150] -> w1099
          frame False {
          }
          frame True {
            n527 = Bundle("wfm info"=w1153, "wfm"=w1152) -> (w1154:T10)  [unwired: 1 in]
            n528 = Set File Position(refnum=w1151, from (0:start)=enum16{"start", "end", "current"}."current", error in=w1156) -> (refnum out=w1160:refnum<file>, error out=w1161:errorcluster)  [unwired: 1 in]
            n529 = Write to Binary File(file (use dialog)=w1160, data=w1154, error in=w1161, 5:FALSE ("prepend array or string size? (T)"), 9:T20."little-endian" ("byte order (0:big-endian, network order)")) -> (refnum out=w1150:refnum<file>, error out=w1155:errorcluster)  [unwired: 1 in, 1 out]
          }
        }
        n530 = Greater?(x=151, y=w1097) -> (0:w1104:bool)
        n531 = case shown="False" w1104 {
          tunnel: [w1120 w1147] -> w1107
          tunnel: w1106 -> [w1121 w1147]
          tunnel: w1103 -> [w1119 w1145]
          tunnel: [w1115 w1145] -> w1105
          tunnel: w1099 -> [w1118 w1146]
          tunnel: w1101 -> [w1117 _]
          tunnel: [w1116 w1146] -> w1098
          tunnel: w1097 -> [_ w1144]
          tunnel: [0 w1143] -> w1096
          frame False {
            n532 = flat-sequence {
              tunnel: w1121 -> [w1131]
              tunnel: [w1131] -> w1124
              tunnel: [w1130] -> w1123
              tunnel: [w1129] -> w1122
              tunnel: w1118 -> [w1129]
              tunnel: w1117 -> [w1127]
              tunnel: w1119 -> [w1126]
              tunnel: [w1125] -> w1115
              tunnel: w1124 -> [w1136]
              tunnel: w1123 -> [w1139]
              tunnel: [w1138] -> w1116
              tunnel: [w1137] -> w1120
              tunnel: w1122 -> [w1135]
              frame #0 {
                n533 = Increment(x=w1126) -> (x+1=w1125:i32)
                n534 = Number To Decimal String(number=w1125) -> (decimal integer string=w1133:string)  [unwired: 1 in]
                n535 = Concatenate Strings("WaveformData_", w1133, ".bin" ("string")) -> (w1132:string)
                n536 = Build Path(base path=w1127, name or relative path=w1132) -> (appended path=w1130:path)
              }
              frame #1 {
                n537 = Close File(refnum=w1135, error in=w1136) -> (error out=w1140:errorcluster)  [unwired: 1 out]
                n538 = Open/Create/Replace File(file path (use dialog)=w1139, error in=w1140, operation (0:open)=T8."open or create", access (0:read/write)=enum16{"read/write", "read-only", "write-only"}."read/write") -> (refnum out=w1138:refnum<file>, error out=w1137:errorcluster)  [unwired: 2 in, 1 out]
              }
            }
          }
          frame True {
            n539 = Increment(x=w1144) -> (x+1=w1143:i32)
          }
        }
      }
    }
    n540 = local read "Exiting"() -> (w793:bool)
    n541 = Less Or Equal To 0?(x=w791) -> (x <= 0?=w794:bool)
    n542 = And(x=w793, y=w794) -> (x .and. y?=w792:bool)
  }
  n543 = while {
    tunnel: w143 -> [w1201]
    shift-right: [w1163] -> w79
    shift-left: w13 -> [w1200]
    tunnel: w8 -> [w1197]
    shift-right: [w1190] -> w88
    shift-left: w61 -> [w1198]
    shift-right: [w1189] -> w87
    shift-left: w58 -> [w1196]
    shift-right: [w1192] -> _
    shift-left: 0 ("binary file indexor in") -> [w1195]
    shift-right: [w1191] -> _
    shift-left: 0 ("binary file indexor in") -> [w1194]
    tunnel: 1000 ("binary file indexor in") -> [w1193]
    tunnel: w142 -> [w1199]
    tunnel: w81 -> [w1169]
    shift-right: [w1178] -> _
    shift-left: FALSE -> [w1177]
    shift-right: [w1174] -> _
    shift-left: 0 -> [w1175]
    shift-right: [w1173] -> _
    shift-left: w82 -> [w1170]
    shift-right: [w1172] -> _
    shift-left: w82 -> [w1171]
    tunnel: "Plot Color Array" -> [w1168]
    stop <- w1186 stop-if-true
    # "If recording data is on, there should always be elements in the queue, so I shouldn't have to worry about a state where the \"recording data\" is active but there is no data in the queue, if so, then I'll just have to find an alternative to the OR statement"
    n544 = Get Queue Status(queue=w1201, error in (no error)=w1200) -> (queue out=w1183:refnum<queue>, error out=w1184:errorcluster, # elements in queue=w1179:i32)  [unwired: 1 in, 5 out]
    n545 = local read "Recording Data"() -> (w1176:bool)
    n546 = Flush Queue(queue=w1183, error in (no error)=w1184) -> (remaining elements=w1182:T15[], error out=w1185:errorcluster)  [unwired: 1 out]
    n547 = Not Equal To 0?(x=w1179) -> (x != 0?=w1181:bool)
    n548 = And(x=w1181, y=w1176) -> (x .and. y?=w1180:bool)
    n549 = case shown="True" w1180 {
      tunnel: w1182 -> [_ w1293]
      tunnel: w1185 -> [w1231 w1287]
      tunnel: w1199 -> [w1232 w1280]
      tunnel: w1198 -> [w1239 w1292]
      tunnel: w1197 -> [w1233 w1291]
      tunnel: w1196 -> [w1240 w1290]
      tunnel: w1195 -> [w1238 w1289]
      tunnel: w1194 -> [w1237 w1279]
      tunnel: w1193 -> [_ w1278]
      tunnel: [w1238 w1286] -> w1192
      tunnel: [w1237 w1285] -> w1191
      tunnel: [w1239 w1282] -> w1190
      tunnel: [w1240 w1281] -> w1189
      tunnel: [w1230 w1272] -> w1167
      tunnel: [w1229 TRUE] -> w1178
      tunnel: w1177 -> [w1228 _]
      tunnel: w1176 -> [w1236 _]
      tunnel: w1175 -> [w1227 w1270]
      tunnel: [w1226 w1269] -> w1174
      tunnel: [w1225 w1276] -> w1173
      tunnel: [w1224 w1273] -> w1172
      tunnel: w1171 -> [w1224 w1268]
      tunnel: w1170 -> [w1225 w1267]
      tunnel: "Time showing on Live Measurements" -> [_ w1261]
      tunnel: w1169 -> [w1223 _]
      tunnel: w1168 -> [w1222 _]
      frame False {
        n550 = Not(x=w1236) -> (.not. x?=w1235:bool)
        n551 = And(x=w1235, y=w1228) -> (x .and. y?=w1234:bool)
        n552 = case shown="True" w1234 {
          tunnel: w1233 -> [_ w1255]
          tunnel: w1232 -> [_ w1254]
          tunnel: w1231 -> [w1243 w1247]
          tunnel: [w1243 w1252] -> w1230
          tunnel: [w1242 FALSE] -> w1229
          tunnel: w1228 -> [w1242 _]
          tunnel: w1227 -> [w1241 _]
          tunnel: [w1241 0] -> w1226
          tunnel: w1223 -> [_ w1245]
          tunnel: w1222 -> [_ w1244]
          frame False {
          }
          frame True {
            n553 = for {
              N: w1245 -> [_]
              shift-right: [w1258] -> w1246
              shift-left: w1247 -> [w1259]
              tunnel: w1244 -> [w1256] mode=indexing
              i -> [w1257]
              n554 = property on="Current Measurements Total" class="XYGraph (strict)"(error in=w1259, "Active Plot"=w1257, "Plot.Plot Color"=w1256) -> (error out=w1260:errorcluster)  [unwired: 1 in, 1 out]
              n555 = property on="Voltage Measurements Total" class="XYGraph (strict)"(error in=w1260, "Active Plot"=w1257, "Plot.Plot Color"=w1256) -> (error out=w1258:errorcluster)  [unwired: 1 in, 1 out]
            }
            n556 = call "ReadDataFile_V1.vi"("error in (no error)"=w1246, "Create CSV files?"=FALSE, "Channel Names Array"=w1254, "DataFolder Path"=w1255) -> ("error out"=w1252:errorcluster, "Current Measurements"=→"Current Measurements Total":cluster{dbl[], dbl[]}[], "Voltage Measurements"=→"Voltage Measurements Total":cluster{dbl[], dbl[]}[])  [unwired: 5 in]
          }
        }
      }
      frame True {
        # "structure where each channel has its own data and supplemental file. Intent for faster data reading speeds in post processing. Probably not since would be i^3, but if we used multiple cores, maybe it would be advantageous"
        n557 = call "FilePathCreation_DCPower_V2.vi"("binary file input reference array 1"=w1292, "Channel Name Input array"=w1280, "data output directory folder"=w1291, "binary file indexor in"=w1289, "Reset counter in"=w1279, "error in (no error)"=w1287, "binary file input reference array 2"=w1290, "reset threshold"=w1278) -> ("binary file output reference array"=w1284:refnum<file>[], "binary file output reference array 2"=w1283:refnum<file>[], "binary file indexor out"=w1286:i32, "reset counter out"=w1285:i32, "error out"=w1288:errorcluster)  [unwired: 3 in]
        n558 = for {
          shift-right: [w1340] -> w1271
          shift-left: w1288 -> [w1341]
          tunnel: w1293 -> [w1350]
          tunnel: w1283 -> [w1347] mode=indexing
          tunnel: w1284 -> [w1346] mode=indexing
          tunnel: [w1345] -> w1281 mode=indexing
          tunnel: [w1339] -> w1282 mode=indexing
          tunnel: [w1328] -> w1275 mode=indexing
          tunnel: [w1327] -> w1274 mode=indexing
          i -> [w1344]
          n559 = for {
            tunnel: w1350 -> [w1363] mode=indexing
            tunnel: w1344 -> [w1360]
            tunnel: [w1355] -> w1335 mode=concatenating
            tunnel: [w1359] -> w1349
            tunnel: w1347 -> [w1358]
            tunnel: w1346 -> [w1356]
            tunnel: [w1356] -> w1342
            tunnel: [w1358] -> w1345
            tunnel: [w1357] -> w1348 mode=concatenating
            n560 = Unbundle(w1363) -> ("Array of fetched data"=w1362:dbl[][][], "Channel Names Array"=w1361:string[])  [unwired: 4 out]
            n561 = Index Array(array=w1361, index=w1360) -> (element=w1359:string)
            n562 = Index Array(array=w1362, index (dim 0)=w1360) -> (element=w1355:dbl[][])  [unwired: 2 in]
            n563 = Array Size(array=w1355) -> (size(s)=w1357:i32[])
          }
          n564 = Bundle("Array of fetched data"=w1335, w1349, w1348) -> (w1343:T21)  [unwired: 1 in]
          n565 = Index Array(array=w1335, index (row)=2) -> (element=w1332:dbl[])  [unwired: 1 in]
          n566 = Index Array(array=w1335, index (row)=1) -> (element=w1333:dbl[])  [unwired: 1 in]
          n567 = Index Array(array=w1335, index (row)=0) -> (element=w1334:dbl[])  [unwired: 1 in]
          n568 = call "DataFileNode_Entry_V4.vi"("error in (no error)"=w1341, "Queued Elements"=w1343, "Byte Stream File in"=w1342) -> ("error out"=w1340:errorcluster, "Byte Stream File out"=w1339:refnum<file>)  [unwired: 7 in]
          n569 = for {
            tunnel: [w1352] -> w1331 mode=indexing if=w1351
            tunnel: w1334 -> [w1352] mode=indexing
            tunnel: [w1354] -> w1329 mode=indexing if=w1351
            tunnel: w1333 -> [w1354] mode=indexing
            tunnel: [w1353] -> w1330 mode=indexing if=w1351
            tunnel: w1332 -> [w1353] mode=indexing
            n570 = Not Equal To 0?(x=w1352) -> (x != 0?=w1351:bool)
          }
          n571 = Bundle(w1331, w1329) -> (w1328:cluster{dbl[], dbl[]})  [unwired: 1 in]
          n572 = Bundle(w1331, w1330) -> (w1327:cluster{dbl[], dbl[]})  [unwired: 1 in]
        }
        n573 = Greater?(x=w1270, y=w1261) -> (0:w1263:bool)
        n574 = Array Size(array=w1267) -> (size(s)=w1266:i32)
        n575 = Equal?(x=w1266, y=0) -> (x = y?=w1264:bool)
        n576 = Or(x=w1263, y=w1264) -> (x .or. y?=w1262:bool)
        n577 = case shown="False" w1262 {
          tunnel: [w1299 w1323] -> w1276
          tunnel: w1267 -> [w1303 _]
          tunnel: w1275 -> [w1302 w1323]
          tunnel: w1268 -> [w1301 _]
          tunnel: w1274 -> [w1300 w1324]
          tunnel: [w1298 w1324] -> w1273
          tunnel: [w1297 w1326] -> w1272
          tunnel: w1271 -> [w1296 w1326]
          tunnel: w1270 -> [w1295 _]
          tunnel: [w1294 0] -> w1269
          frame False {
            n578 = for {
              tunnel: w1303 -> [w1322] mode=indexing
              tunnel: w1302 -> [w1319] mode=indexing
              tunnel: w1301 -> [w1316] mode=indexing
              tunnel: w1300 -> [w1315] mode=indexing
              tunnel: [w1306] -> w1299 mode=indexing
              tunnel: [w1305] -> w1298 mode=indexing
              shift-right: [w1304] -> w1297
              shift-left: w1296 -> [w1304]
              n579 = Unbundle(w1322) -> (w1321:dbl[], w1320:dbl[])
              n580 = Unbundle(w1319) -> (w1318:dbl[], w1317:dbl[])
              n581 = Unbundle(w1316) -> (w1314:dbl[], w1313:dbl[])
              n582 = Unbundle(w1315) -> (w1312:dbl[], w1311:dbl[])
              n583 = Insert Into Array(array=w1314, new element=w1312) -> (w1309:dbl[])  [unwired: 1 in]
              n584 = Insert Into Array(array=w1321, new element=w1318) -> (w1307:dbl[])  [unwired: 1 in]
              n585 = Insert Into Array(array=w1313, new element=w1311) -> (w1310:dbl[])  [unwired: 1 in]
              n586 = Insert Into Array(array=w1320, new element=w1317) -> (w1308:dbl[])  [unwired: 1 in]
              n587 = Bundle(w1309, w1310) -> (w1305:cluster{dbl[], dbl[]})  [unwired: 1 in]
              n588 = Bundle(w1307, w1308) -> (w1306:cluster{dbl[], dbl[]})  [unwired: 1 in]
            }
            n589 = Increment(x=w1295) -> (x+1=w1294:i32)
          }
          frame True {
          }
        }
        "Voltage Measurements Live" <- w1276
        "Current Measurements Live" <- w1273
      }
    }
    n590 = Equal To 0?(x=w1179) -> (x = 0?=w1187:bool)
    n591 = case shown="True" "Live Measurement Range Update" {
      tunnel: w1167 -> [w1212 w1221]
      tunnel: [w1212 w1220] -> w1164
      frame False {
      }
      frame True {
        (unwired) 0.001 ("Delay Time (s)")
        n592 = property on="Voltage Measurements Live" class="XYGraph (strict)"(error in=w1221, "YScale.Maximum"="Live Voltage Y Max", "YScale.Minimum"="Live Voltage Y Min") -> (error out=w1214:errorcluster)  [unwired: 1 in, 1 out]
        n593 = property on="Current Measurements Live" class="XYGraph (strict)"(error in=w1214, "ActXScl"=0 ("Active X Scale")) -> (error out=w1213:errorcluster)  [unwired: 1 in, 1 out]
        n594 = property on="Current Measurements Live" class="XYGraph (strict)"(error in=w1213, "YScale.Maximum"="Live Current Y Max", "YScale.Minimum"="Live Current Y Min") -> (error out=w1220:errorcluster)  [unwired: 1 in, 1 out]
      }
    }
    n595 = local read "Exiting"() -> (w1188:bool)
    n596 = And(x=w1187, y=w1188) -> (x .and. y?=w1186:bool)
    n597 = case shown="True" "Total Measurement Range Update" {
      tunnel: w1164 -> [w1202 w1211]
      tunnel: [w1202 w1209] -> w1163
      frame False {
      }
      frame True {
        n598 = property on="Voltage Measurements Total" class="XYGraph (strict)"(error in=w1211, "YScale.Maximum"="Total Voltage Y Max", "YScale.Minimum"="Total Voltage Y Min", "XScale.Maximum"="Total Time X Max", "XScale.Minimum"="Total Time X Min") -> (error out=w1210:errorcluster)  [unwired: 1 in, 1 out]
        n599 = property on="Current Measurements Total" class="XYGraph (strict)"(error in=w1210, "YScale.Maximum"="Total Current Y Max", "YScale.Minimum"="Total Current Y Min", "XScale.Maximum"="Total Time X Max", "XScale.Minimum"="Total Time X Min") -> (error out=w1209:errorcluster)  [unwired: 1 in, 1 out]
      }
    }
  }
  n600 = Strip Path(path=w8) -> (stripped path=w7:path)  [unwired: 1 out]
  n601 = Build Path(base path=w7, name or relative path="ResetTimeStamps.csv") -> (appended path=w5:path)
  n602 = while {
    shift-right: [w1406] -> w152
    shift-left: "DCPowerInformationClusterArray_Input" -> [w1406]
    shift-right: [w1409] -> w153
    shift-left: "VISAPowerInfoInputArray" -> [w1409]
    shift-right: [w1408] -> w154
    shift-left: w147 -> [w1408]
    shift-right: [w1407] -> w156
    shift-left: "RF Block Input Array" -> [w1407]
    shift-right: [w1380] -> w75
    shift-left: w68 -> [w1405]
    tunnel: w132 -> [w1378]
    shift-right: [w1404] -> _
    shift-left: FALSE -> [w1401]
    tunnel: w143 -> [w1403]
    shift-right: [w1388] -> _
    shift-left: FALSE -> [w1393]
    tunnel: [w1397] -> w93
    shift-right: [w1391] -> _
    shift-left: TRUE ("x .and. y?") -> [w1392]
    shift-right: [w1389] -> _
    shift-left: w84 -> [w1390]
    tunnel: [w1388] -> w151
    tunnel: w161 -> [w1386]
    shift-right: [w1375] -> _
    shift-left: TRUE -> [w1374]
    tunnel: w69 -> [w1370]
    tunnel: [w1369] -> w76
    shift-right: [w1366] -> _
    shift-left: FALSE ("x") -> [w1368]
    tunnel: w7 -> [w1367]
    tunnel: w5 -> [w1365]
    stop <- w1387 stop-if-true
    # "If I am going to reset the entire configuration or if we are going up in LET only. True, reset the system. False, don't reset the system"
    n603 = Not(x=w1393) -> (.not. x?=w1395:bool)
    n604 = And(x="Record Data Toggle", y=w1395) -> (x .and. y?=w1396:bool)
    "Recording Data" <- w1396
    n605 = case shown="True" w1396 {
      tunnel: w1378 -> [w1490 w1501]
      tunnel: w1405 -> [w1488 w1533]
      tunnel: [w1479 w1527] -> w1385
      tunnel: [w1480 w1526] -> w1384
      tunnel: w1401 -> [_ w1531]
      tunnel: [FALSE w1532] -> w1404
      tunnel: w1403 -> [_ w1530]
      tunnel: [w1478 w1529] -> w1373
      tunnel: "Record Data Toggle" -> [w1486 _]
      tunnel: w1393 -> [w1487 _]
      tunnel: w1392 -> [w1482 _]
      tunnel: [w1483 TRUE] -> w1391
      tunnel: w1390 -> [w1481 w1534]
      tunnel: [w1481 w1507] -> w1389
      tunnel: w1386 -> [_ w1525]
      tunnel: w1370 -> [w1477 w1521]
      tunnel: [w1477 w1524] -> w1369
      tunnel: w1368 -> [w1476 w1515]
      tunnel: w1367 -> [_ w1511]
      tunnel: [w1476 w1512] -> w1366
      tunnel: w1365 -> [_ w1506]
      tunnel: "Software Mitigation?" -> [_ w1500]
      frame False {
        n606 = And(x=w1486, y=w1487) -> (x .and. y?=w1485:bool)
        n607 = And(x=w1482, y=w1485) -> (x .and. y?=w1484:bool)
        n608 = case shown="True" w1484 {
          tunnel: [w1492 w1494] -> w1475
          tunnel: w1488 -> [w1492 w1495]
          tunnel: [w1491 FALSE] -> w1483
          tunnel: w1482 -> [w1491 _]
          frame False {
          }
          frame True {
            n609 = call "Display Message to User2"("error in (no error)"=w1495) -> ("error out"=w1494:errorcluster)  [unwired: 9 in, 1 out]
          }
        }
        n610 = call "Fetch&Process_Measurements_V4.vi"("DCPowerInformationArrayOutput_byChannel"=w1490, "Initial Time"=w1481, "error in (no error)"=w1475) -> ("Current Waveform Array"=w1479:waveform(dbl)[], "Voltage Waveform Array"=w1480:waveform(dbl)[], "error out"=w1478:errorcluster)  [unwired: 4 in, 6 out]
      }
      frame True {
        n611 = case shown="False" w1531 {
          tunnel: [w1589 w1609] -> w1507
          tunnel: w1534 -> [_ w1609]
          tunnel: w1533 -> [w1591 w1608]
          tunnel: [w1590 w1608] -> w1520
          tunnel: [TRUE w1607] -> w1532
          tunnel: w1531 -> [_ w1607]
          tunnel: w1511 -> [w1588 _]
          frame False {
            n612 = Get Date/Time In Seconds() -> (seconds since 1Jan1904=w1589:timestamp)
            n613 = Get Date/Time String(date format (0)=enum16{"short", "long", "abbreviated"}."short", seconds (now)=w1589, want seconds? (F)=TRUE) -> (date string=w1603:string, time string=w1604:string)
            n614 = Concatenate Strings(w1603, "_" ("string"), w1604) -> (w1602:string)
            n615 = Build Path(base path=w1588, name or relative path="BeginRecordTimeStamp.txt") -> (appended path=w1598:path)
            n616 = Open/Create/Replace File(file path (use dialog)=w1598, error in=w1591, operation (0:open)=T8."open or create", access (0:read/write)=enum16{"read/write", "read-only", "write-only"}."read/write") -> (refnum out=w1601:refnum<file>, error out=w1605:errorcluster)  [unwired: 2 in, 1 out]
            n617 = Write to Text File(file (use dialog)=w1601, text=w1602, error in=w1605) -> (refnum out=w1599:refnum<file>, error out=w1600:errorcluster)  [unwired: 1 in, 1 out]
            n618 = Close File(refnum=w1599, error in=w1600) -> (error out=w1590:errorcluster)  [unwired: 1 out]
          }
          frame True {
          }
        }
        n619 = call <instrlib>:"niDMM Initiate.vi"("error in (no error)"=w1520, "instrument handle"=w1521) -> ("error out"=w1523:errorcluster, "instrument handle out"=w1522:refnum<k15>)  [unwired: 8 in]
        n620 = call <instrlib>:"niDMM Fetch.vi"("error in (no error)"=w1523, "instrument handle"=w1522) -> ("error out"=w1514:errorcluster, "Measurement"=w1519:dbl, "instrument handle out"=w1524:refnum<k15>)  [unwired: 7 in]
        "Measurement" <- w1519
        n621 = Greater?(x=w1519, y=3.0) -> (0:w1516:bool)
        n622 = Exclusive Or(1:w1516, 2:w1515) -> (0:w1517:bool)
        n623 = case shown="True" w1517 {
          tunnel: w1515 -> [w1562 w1583]
          tunnel: w1511 -> [_ w1564]
          tunnel: w1514 -> [w1563 w1580]
          tunnel: [w1563 w1566] -> w1513
          tunnel: [w1562 w1565] -> w1512
          frame False {
          }
          frame True {
            n624 = case shown="False" w1583 {
              tunnel: ["BeamStartTime.txt" "BeamEndTime.txt"] -> w1582
              tunnel: [TRUE FALSE] -> w1565
              frame False {
              }
              frame True {
              }
            }
            n625 = Build Path(base path=w1564, name or relative path=w1582) -> (appended path=w1581:path)
            n626 = Open/Create/Replace File(file path (use dialog)=w1581, error in=w1580, operation (0:open)=T8."open or create", access (0:read/write)=enum16{"read/write", "read-only", "write-only"}."read/write") -> (refnum out=w1570:refnum<file>, error out=w1569:errorcluster)  [unwired: 2 in, 1 out]
            n627 = Get Date/Time In Seconds() -> (seconds since 1Jan1904=w1577:timestamp)
            n628 = Get Date/Time String(date format (0)=enum16{"short", "long", "abbreviated"}."short", seconds (now)=w1577, want seconds? (F)=TRUE) -> (date string=w1575:string, time string=w1576:string)
            n629 = Concatenate Strings(w1575, "_" ("string"), w1576) -> (w1571:string)
            n630 = Write to Text File(file (use dialog)=w1570, text=w1571, error in=w1569) -> (refnum out=w1567:refnum<file>, error out=w1568:errorcluster)  [unwired: 1 in, 1 out]
            n631 = Close File(refnum=w1567, error in=w1568) -> (error out=w1566:errorcluster)  [unwired: 1 out]
          }
        }
        n632 = call "Fetch&Process_Measurements_V4.vi"("DCPowerInformationArrayOutput_byChannel"=w1501, "Initial Time"=w1507, "error in (no error)"=w1513) -> ("Current Reading too High?"=w1505:bool[], "Data As dbl Array"=w1510:dbl[][][], "Channel Number Array"=w1504:string[], "Current Waveform Array"=w1527:waveform(dbl)[], "Voltage Waveform Array"=w1526:waveform(dbl)[], "Current Reading Indices"=w1503:i32[], "TimeStampArrayDouble"=w1502:dbl[], "error out"=w1509:errorcluster)  [unwired: 4 in, 1 out]
        n633 = Or Array Elements(Boolean array=w1505) -> (logical OR=w1499:bool)
        n634 = Bundle(cluster=w1525, "Array of fetched data"=w1510, "Channel Names Array"=w1504, "Beam Logic"=w1519) -> (w1528:T15)  [unwired: 3 in]
        n635 = And(x=w1500, y=w1499) -> (x .and. y?=w1498:bool)
        n636 = Or(x="User Forced Reset", y=w1498) -> (x .or. y?=w1497:bool)
        n637 = case shown="True" w1497 {
          tunnel: w1509 -> [w1536 w1546]
          tunnel: [w1536 w1543] -> w1508
          tunnel: w1507 -> [_ _]
          tunnel: w1506 -> [_ w1559]
          tunnel: w1505 -> [_ w1555]
          tunnel: w1504 -> [_ w1554]
          tunnel: w1503 -> [_ _]
          tunnel: w1502 -> [_ w1551]
          tunnel: w1501 -> [_ w1542]
          tunnel: "User Forced Reset" -> [_ w1539]
          frame False {
          }
          frame True {
            w1540 = i32[] [1]  # DCPower_ToggleIndex
            n638 = Search 1D Array(1D array=w1555, element=TRUE) -> (index of element=w1550:i32)  [unwired: 1 in]
            n639 = Index Array(array=w1551, index=w1550) -> (element=w1549:dbl)
            n640 = Index Array(array=w1554, index=w1550) -> (element=w1552:string)
            n641 = Boolean To (0,1)(Boolean=w1539) -> (0, 1=w1538:i16)
            n642 = Number To Fractional String(number=w1549) -> (F-format string=w1553:string)  [unwired: 3 in]
            n643 = Number To Decimal String(number=w1538) -> (decimal integer string=w1537:string)  [unwired: 1 in]
            n644 = call "DCPower_TurnOff_byIndividualChannel_KeepReference.vi"("error in (no error)"=w1546, "DCPower_ToggleIndex"=w1540, "DCPower_byChannel in"=w1542) -> ("error out"=w1545:errorcluster, "DCPower_byChannel out"=w1541:T16)
            n645 = Build Array(w1553, w1552, w1537) -> (w1557:string[])
            n646 = call-poly <vilib>:"Write Delimited Spreadsheet.vi"("file path (dialog if empty)"=w1559, "format (%s)"="%s" ("format (%.3f)"), "1D data"=w1557, "append to file? (new file:F)"=TRUE, "error in (no error)"=w1545, "delimiter (\\t)"="," ("delimiter (\\t)")) -> ("error out"=w1548:errorcluster)  [unwired: 8 in, 1 out]
            n647 = call "Time Delay"("error in (no error)"=w1548, "Delay Time (s)"=0.1) -> ("error out"=w1544:errorcluster)  [unwired: 9 in]
            n648 = call "DCPower_Reconfig_byChannel.vi"("error in (no error)"=w1544, "DCPower_ToggleIndex"=w1540, "DCPower_byChannel in 2"=w1541) -> ("error out"=w1543:errorcluster)  [unwired: 1 out]
          }
        }
        n649 = Enqueue Element(queue=w1530, element=w1528, error in (no error)=w1508) -> (error out=w1529:errorcluster)  [unwired: 1 in, 2 out]
      }
    }
    "Current Waveform Array" <- w1385
    "Voltage Waveform Array" <- w1384
    n650 = Not(x=w1396) -> (.not. x?=w1402:bool)
    n651 = And(x=w1402, y=w1401) -> (x .and. y?=w1400:bool)
    n652 = case shown="True" "Waveform Update" {
      tunnel: [w1410 w1419] -> w1372
      tunnel: w1373 -> [w1410 w1416]
      frame False {
      }
      frame True {
        n653 = property on="Voltage Waveform Array" class="WFChart (strict)"(error in=w1416, "ActYScl"=0 ("Active Y Scale")) -> (error out=w1415:errorcluster)  [unwired: 1 in, 1 out]
        n654 = property on="Voltage Waveform Array" class="WFChart (strict)"(error in=w1415, "YScale.Maximum"="Voltage Waveform Y Max", "YScale.Minimum"="Voltage Waveform Y Min") -> (error out=w1414:errorcluster)  [unwired: 1 in, 1 out]
        n655 = property on="Current Waveform Array" class="WFChart (strict)"(error in=w1414, "ActYScl"=0 ("Active Y Scale")) -> (error out=w1413:errorcluster)  [unwired: 1 in, 1 out]
        n656 = property on="Current Waveform Array" class="WFChart (strict)"(error in=w1413, "YScale.Maximum"="Current Waveform Y Max", "YScale.Minimum"="Current Waveform Y Min") -> (error out=w1419:errorcluster)  [unwired: 1 in, 1 out]
      }
    }
    n657 = Exclusive Or(1:"Device Powered?", 2:w1374) -> (0:w1377:bool)
    n658 = case shown="True" w1377 {
      tunnel: [w1423 w1427] -> w1379
      tunnel: w1372 -> [w1423 w1426]
      tunnel: w1378 -> [_ w1428]
      tunnel: "Device Powered?" -> [w1422 w1425]
      tunnel: [w1422 w1424] -> w1375
      frame False {
      }
      frame True {
        n659 = case shown="True" w1425 {
          selector: w1425 -> [w1429 w1445]
          tunnel: w1428 -> [w1432 w1448]
          tunnel: [w1430 w1447] -> w1427
          tunnel: w1426 -> [w1431 w1446]
          tunnel: [w1429 w1445] -> w1424
          frame False {
            n660 = for {
              tunnel: w1432 -> [w1444] mode=indexing
              shift-right: [w1434] -> w1430
              shift-left: w1431 -> [w1435]
              n661 = Unbundle(w1444) -> ("IVI Refnum out"=w1443:refnum<k15>, w1436:string)  [unwired: 7 out]
              n662 = call <instrlib>:"niDCPower Abort With Channels.vi"("error in (no error)"=w1435, "channel name"=w1436, "instrument handle"=w1443) -> ("error out"=w1442:errorcluster, "instrument handle out"=w1441:refnum<k15>)  [unwired: 7 in]
              n663 = call <instrlib>:"niDCPower Configure Voltage Level.vi"("error in (no error)"=w1442, "voltage level"=0.0, "channel name"=w1436, "instrument handle"=w1441) -> ("error out"=w1440:errorcluster, "instrument handle out"=w1439:refnum<k15>)  [unwired: 6 in]
              n664 = call <instrlib>:"niDCPower Commit With Channels.vi"("error in (no error)"=w1440, "channel name"=w1436, "instrument handle"=w1439) -> ("error out"=w1438:errorcluster, "instrument handle out"=w1437:refnum<k15>)  [unwired: 7 in]
              n665 = call <instrlib>:"niDCPower Initiate With Channels.vi"("error in (no error)"=w1438, "channel name"=w1436, "instrument handle"=w1437) -> ("error out"=w1434:errorcluster)  [unwired: 7 in, 1 out]
            }
          }
          frame True {
            n666 = for {
              tunnel: w1448 -> [w1460] mode=indexing
              shift-right: [w1450] -> w1447
              shift-left: w1446 -> [w1451]
              n667 = Unbundle(w1460) -> ("IVI Refnum out"=w1459:refnum<k15>, w1452:string, "voltage level channel 23"=w1449:dbl)  [unwired: 6 out]
              n668 = call <instrlib>:"niDCPower Abort With Channels.vi"("error in (no error)"=w1451, "channel name"=w1452, "instrument handle"=w1459) -> ("error out"=w1458:errorcluster, "instrument handle out"=w1457:refnum<k15>)  [unwired: 7 in]
              n669 = call <instrlib>:"niDCPower Configure Voltage Level.vi"("error in (no error)"=w1458, "voltage level"=w1449, "channel name"=w1452, "instrument handle"=w1457) -> ("error out"=w1456:errorcluster, "instrument handle out"=w1455:refnum<k15>)  [unwired: 6 in]
              n670 = call <instrlib>:"niDCPower Commit With Channels.vi"("error in (no error)"=w1456, "channel name"=w1452, "instrument handle"=w1455) -> ("error out"=w1454:errorcluster, "instrument handle out"=w1453:refnum<k15>)  [unwired: 7 in]
              n671 = call <instrlib>:"niDCPower Initiate With Channels.vi"("error in (no error)"=w1454, "channel name"=w1452, "instrument handle"=w1453) -> ("error out"=w1450:errorcluster)  [unwired: 7 in, 1 out]
            }
          }
        }
      }
    }
    n672 = case shown="True" w1400 {
      tunnel: w1379 -> [w1471 w1473]
      tunnel: [w1472 TRUE] -> w1388
      tunnel: w1393 -> [w1472 _]
      tunnel: [w1471 w1473] -> w1380
      frame False {
      }
      frame True {
      }
    }
    "error of collection" <- w1380
    "Ready For Next Run?" <- w1388
    n673 = And(x="Next Run", y=w1388) -> (x .and. y?=w1399:bool)
    n674 = Or(x="force exit SubVI", y=w1399) -> (x .or. y?=w1382:bool)
    n675 = Or(x=w1380, y=w1382) -> (x .or. y?=w1381:bool)
    n676 = case shown="True" w1381 {
      selector: w1381 -> [w1462 _]
      tunnel: w1380 -> [_ w1465]
      tunnel: [w1462 TRUE] -> w1387
      tunnel: [TRUE ("T button?") w1463] -> w1397
      frame False {
        # "Don't end the run"
      }
      frame True {
        n677 = case shown="No Error" w1465 {
          tunnel: [w1466 TRUE] -> w1463
          frame No Error {
            # "Option to continue the run as is or reset for a new configuration"
            n678 = Two Button Dialog(message="Would you like to change parameters before the next run? ( you will have an option to change LET and board number regardless) ", 1:"No, I may only want to change LET or board number" ("F button name (\"Cancel\")"), 2:"Yes, I want to make changes " ("T button name (\"OK\")")) -> (T button?=w1466:bool)
          }
          frame Error {
            # "End the run immediately. There is an error or an immediate issue with the VI"
          }
        }
      }
    }
    "Exiting" <- w1387
  }
  "Reinitialize?" <- w93
  n679 = Merge Errors(w79) -> (w80:errorcluster)
  n680 = for {
    tunnel: w88 -> [w1614] mode=indexing
    tunnel: w87 -> [w1612] mode=indexing
    shift-right: [w1610] -> w160
    shift-left: w80 -> [w1613]
    n681 = Close File(refnum=w1614, error in=w1613) -> (error out=w1611:errorcluster)  [unwired: 1 out]
    n682 = disable-structure shown="Enabled" {
      disable-tunnel: w1612 -> [w1618 _]
      disable-tunnel: w1611 -> [w1617 w1619]
      disable-tunnel: [w1616 w1619] -> w1610
      frame Enabled {
        n683 = Close File(refnum=w1618, error in=w1617) -> (error out=w1616:errorcluster)  [unwired: 1 out]
      }
      frame Disabled {
      }
    }
    n684 = case shown="Error .." w1610 {
      selector: w1610 -> [_ w1615]
      frame No Error {
      }
      frame Error {
        "error IO" <- w1615
      }
    }
  }
  n685 = Close File(refnum=w45, error in=w42) -> (error out=w41:errorcluster)  [unwired: 1 out]
  n686 = for {
    tunnel: w43 -> [w1622] mode=indexing
    shift-right: [w1621] -> w1
    shift-left: w41 -> [w1620]
    n687 = Close File(refnum=w1622, error in=w1620) -> (error out=w1621:errorcluster)  [unwired: 1 out]
  }
  n688 = call <instrlib>:"niDMM Close.vi"("error in (no error)"=w75, "instrument handle"=w76) -> ("error out"=w162:errorcluster)  [unwired: 9 in]
  n689 = Merge Errors(w20, w1) -> (w21:errorcluster)
  n690 = call <instrlib>:"niScope Close.vi"("instrument handle"=w17, "error in"=w21) -> ("error out"=w120:errorcluster)  [unwired: 13 in]
  n691 = Merge Errors(w162, w160, w120) -> (w159:errorcluster)
  n692 = Unbundle(w158) -> ("created path"=w96:path)  [unwired: 2 out]
  n693 = Strip Path(path=w96) -> (stripped path=w95:path)  [unwired: 1 out]
  n694 = case shown="True" w151 {
    selector: w151 -> [w1629 w1756]
    tunnel: w159 -> [w1624 w1762]
    tunnel: [w1633 w1694] -> w136
    tunnel: "Oscilloscope Configuration Input Array" -> [w1633 w1761]
    tunnel: [w1632 w1696] -> w157
    tunnel: w156 -> [w1632 w1760]
    tunnel: [w1631 w1682] -> w155
    tunnel: w154 -> [w1631 w1759]
    tunnel: [w1630 w1699] -> w121
    tunnel: w153 -> [w1630 w1758]
    tunnel: [w1625 w1701] -> w9
    tunnel: w152 -> [w1625 w1757]
    tunnel: [w1629 w1756] -> w150
    tunnel: [string[][] [] ("DCPowerInfoArray") w1692] -> w149
    tunnel: w95 -> [_ w1648]
    tunnel: [string[][] [] ("DCPowerInfoArray") w1690] -> w137
    tunnel: [string[][] [] ("DCPowerInfoArray") w1684] -> w145
    tunnel: [w1623 w1643] -> w138
    frame False {
      (unwired) string[][][] []
      n695 = for {
        tunnel: w1625 -> [w1636] mode=indexing
        shift-right: [w1637] -> w1623
        shift-left: w1624 -> [w1638]
        n696 = Unbundle(w1636) -> ("IVI Refnum out"=w1635:refnum<k15>, "Active Channel Numbers String List"=w1634:string)  [unwired: 8 out]
        n697 = call <instrlib>:"niDCPower Abort With Channels.vi"("error in (no error)"=w1638, "channel name"=w1634, "instrument handle"=w1635) -> ("error out"=w1637:errorcluster)  [unwired: 7 in, 1 out]
      }
    }
    frame True {
      # "This will be indexed eventually"
      n698 = for {
        shift-right: [w1873] -> w1653
        shift-left: w1762 -> [w1884]
        tunnel: w1757 -> [w1871] mode=indexing
        shift-right: [w1883] -> w1732
        shift-left: w1761 -> [w1883]
        shift-right: [w1882] -> w1731
        shift-left: w1760 -> [w1882]
        shift-right: [w1881] -> w1730
        shift-left: w1759 -> [w1881]
        shift-right: [w1880] -> w1729
        shift-left: w1758 -> [w1880]
        shift-right: [w1879] -> w1728
        shift-left: w1757 -> [w1879]
        shift-right: [w1877] -> w1733
        shift-left: string[][] [] ("DCPowerInfoArray") -> [w1878]
        # "This puts all the instruments together in one output"
        n699 = Unbundle(w1871) -> ("IVI Refnum out"=w1886:refnum<k15>, "Active Channel Numbers String List"=w1885:string)  [unwired: 8 out]
        n700 = call <instrlib>:"niDCPower Abort With Channels.vi"("error in (no error)"=w1884, "channel name"=w1885, "instrument handle"=w1886) -> ("error out"=w1874:errorcluster)  [unwired: 7 in, 1 out]
        n701 = call "DCPower_ParameterCreation.vi"("error in"=w1874, "Precision"="8", "DCPowerInformationByInstrument"=w1871) -> ("error out"=w1873:errorcluster, "DCPowerInfoArray"=w1872:string[][])
        n702 = Insert Into Array(array=w1878, index (col)=0 ("disabled index (col)"), new element=w1872) -> (w1877:string[][])  [unwired: 1 in]
      }
      n703 = Concatenate Strings("Aperture Time (s)" ("element")) -> (w1651:string)
      n704 = Concatenate Strings("Channel Name " ("string")) -> (w1745:string)
      n705 = Concatenate Strings("Voltage (V) " ("string")) -> (w1747:string)
      n706 = Concatenate Strings("Measure Record delta Time (s) " ("string")) -> (w1749:string)
      n707 = Concatenate Strings("Instrument Name " ("string")) -> (w1744:string)
      n708 = Concatenate Strings("Instrument Channel Number " ("string")) -> (w1746:string)
      n709 = Concatenate Strings("Current Clamp (A) " ("string")) -> (w1748:string)
      n710 = Build Array(w1744, w1745, w1746, w1747, w1748, w1749, w1651, "Current Reset Value (A)") -> (w1737:string[])
      n711 = Build Path(base path=w1648, name or relative path="DCPOW_Params.csv") -> (appended path=w1752:path)
      n712 = Insert Into Array(array=w1733, index (col)=0 ("disabled index (col)"), new element=w1737) -> (w1736:string[][])  [unwired: 1 in]
      n713 = call-poly <vilib>:"Write Delimited Spreadsheet.vi"("file path (dialog if empty)"=w1752, "format (%s)"="%s" ("format (%.3f)"), "2D data"=w1736, "error in (no error)"=w1653, "transpose? (no:F)"=TRUE, "delimiter (\\t)"="," ("delimiter (\\t)")) -> ("error out"=w1734:errorcluster)  [unwired: 8 in, 1 out]
      n714 = for {
        shift-right: [w1865] -> w1714
        shift-left: w1734 -> [w1865]
        shift-right: [w1860] -> w1702
        shift-left: w1728 -> [w1860]
        shift-right: [w1861] -> w1700
        shift-left: w1729 -> [w1861]
        shift-right: [w1862] -> w1698
        shift-left: w1730 -> [w1862]
        shift-right: [w1863] -> w1697
        shift-left: w1731 -> [w1863]
        shift-right: [w1864] -> w1693
        shift-left: w1733 -> [w1864]
        tunnel: w1732 -> [w1859] mode=indexing
        tunnel: [w1859] -> w1695 mode=indexing
        shift-right: [w1828] -> w1691
        shift-left: string[][] [] ("DCPowerInfoArray") -> [w1834]
        n715 = Unbundle(w1859) -> ("Instrument Reference"=w1858:refnum<k15>, "active channel number string array"=w1831:string[], "active channel names array"=w1832:string[], "1M ohm vertical range"=w1853:dbl, "vertical coupling"=w1847:T3, "Channel 0 50 ohms?"=w1852:bool, "50 ohm vertical range (V)"=w1851:dbl, "min record length"=w1846:i32, "Actual Sample Rate"=w1845:dbl)  [unwired: 1 out]
        n716 = Array Size(array=w1831) -> (size(s)=w1854:i32)
        n717 = Initialize Array(w1853, w1854) -> (w1850:dbl[])
        n718 = Decimal String To Number(string="8") -> (number=w1829:i32)  [unwired: 2 in, 1 out]
        n719 = case shown="True" w1852 {
          tunnel: w1851 -> [_ w1868]
          tunnel: w1850 -> [w1866 w1870]
          tunnel: [w1866 w1867] -> w1849
          frame False {
          }
          frame True {
            n720 = Replace Array Subset(array=w1870, new element=w1868, index=0) -> (w1867:dbl[])
          }
        }
        n721 = Number To Fractional String(number=w1845, precision (6)=w1829) -> (F-format string=w1839:string)  [unwired: 2 in]
        n722 = Number To Decimal String(number=w1846) -> (decimal integer string=w1840:string)  [unwired: 1 in]
        n723 = Concatenate Strings(w1858) -> (w1856:string)
        n724 = Number To Fractional String(number=w1849, precision (6)=w1829) -> (F-format string=w1848:string[])  [unwired: 2 in]
        n725 = Number To Decimal String(number=w1847) -> (decimal integer string=w1841:string)  [unwired: 1 in]
        n726 = Array Size(array=w1831) -> (size(s)=w1857:i32)
        n727 = Initialize Array(w1856, w1857) -> (w1855:string[])
        n728 = Array Size(array=w1831) -> (size(s)=w1844:i32)
        n729 = Array Size(array=w1831) -> (size(s)=w1842:i32)
        n730 = Array Size(array=w1831) -> (size(s)=w1843:i32)
        n731 = Initialize Array(w1841, w1844) -> (w1838:string[])
        n732 = Initialize Array(w1839, w1842) -> (w1836:string[])
        n733 = Initialize Array(w1840, w1843) -> (w1837:string[])
        n734 = Build Array(w1855, w1832, w1831, w1848, w1838, w1837, w1836) -> (w1833:string[][])
        n735 = Insert Into Array(array=w1834, index (col)=0 ("disabled index (col)"), new element=w1833) -> (w1828:string[][])  [unwired: 1 in]
      }
      n736 = Build Array("Instrument Name " ("string"), "Channel Name" ("element"), "Instrument Channel Number" ("element"), "Vertical Range (V)" ("element"), "Vertical Coupling" ("element"), "Min Record Length" ("element"), "Actual Sample Rate" ("element")) -> (w1718:string[])
      n737 = Insert Into Array(array=w1691, index (col)=0 ("disabled index (col)"), new element=w1718) -> (w1711:string[][])  [unwired: 1 in]
      n738 = Build Path(base path=w1648, name or relative path="Oscilloscope_Params.csv") -> (appended path=w1716:path)
      n739 = call-poly <vilib>:"Write Delimited Spreadsheet.vi"("file path (dialog if empty)"=w1716, "format (%s)"="%s" ("format (%.3f)"), "2D data"=w1711, "error in (no error)"=w1714, "transpose? (no:F)"=TRUE, "delimiter (\\t)"="," ("delimiter (\\t)")) -> ("error out"=w1709:errorcluster)  [unwired: 8 in, 1 out]
      n740 = for {
        shift-right: [w1810] -> w1707
        shift-left: string[][] [] ("DCPowerInfoArray") -> [w1811]
        tunnel: w1697 -> [w1826] mode=indexing
        shift-right: [w1795] -> w1683
        shift-left: w1709 -> [w1802]
        shift-right: [w1803] -> w1690
        shift-left: w1691 -> [w1803]
        shift-right: [w1804] -> w1692
        shift-left: w1693 -> [w1804]
        shift-right: [w1805] -> w1694
        shift-left: w1695 -> [w1805]
        shift-right: [w1806] -> w1696
        shift-left: w1697 -> [w1806]
        shift-right: [w1807] -> w1682
        shift-left: w1698 -> [w1807]
        shift-right: [w1808] -> w1699
        shift-left: w1700 -> [w1808]
        shift-right: [w1809] -> w1701
        shift-left: w1702 -> [w1809]
        n741 = Unbundle(w1826) -> ("VISA resource name"=w1825:refnum<visa-resource-name>, "Frequency (GHz) Output"=w1819:dbl, "Power (dBm) Output"=w1816:dbl)  [unwired: 2 out]
        n742 = Decimal String To Number(string="8") -> (number=w1814:i32)  [unwired: 2 in, 1 out]
        n743 = VISA Write(VISA resource name=w1825, write buffer="*IDN?", error in (no error)=w1802) -> (VISA resource name out=w1821:refnum<visa-resource-name>, return count=w1823:u32, error out=w1827:errorcluster)
        n744 = Number To Fractional String(number=w1816, precision (6)=w1814) -> (F-format string=w1817:string)  [unwired: 2 in]
        n745 = Add(x=w1823, y=u32 10) -> (x+y=w1820:u32)
        n746 = Number To Fractional String(number=w1819, precision (6)=w1814) -> (F-format string=w1818:string)  [unwired: 2 in]
        n747 = VISA Read(VISA resource name=w1821, byte count=w1820, error in (no error)=w1827) -> (read buffer=w1801:string, error out=w1796:errorcluster)  [unwired: 2 out]
        n748 = Search and Replace String(replace all?=TRUE ("replace all? (F)"), input string=w1801, search string=",", replace string="_" ("replace string (\"\")"), error in=w1796) -> (result string=w1798:string, error out=w1795:errorcluster)  [unwired: 3 in, 2 out]
        n749 = Build Array(w1798, w1818, w1817) -> (w1813:string[])
        n750 = Insert Into Array(array=w1811, index (col)=0 ("index (row)"), new element=w1813) -> (w1810:string[][])  [unwired: 1 in]
      }
      n751 = Build Array("Instrument Name", "Frequency (GHz)" ("element"), "Power (dBm)" ("element")) -> (w1703:string[])
      n752 = Build Path(base path=w1648, name or relative path="RFSource_Params.csv") -> (appended path=w1688:path)
      n753 = Insert Into Array(array=w1707, index (col)=0 ("disabled index (col)"), new element=w1703) -> (w1684:string[][])  [unwired: 1 in]
      n754 = call-poly <vilib>:"Write Delimited Spreadsheet.vi"("file path (dialog if empty)"=w1688, "format (%s)"="%s" ("format (%.3f)"), "2D data"=w1684, "error in (no error)"=w1683, "transpose? (no:F)"=TRUE, "delimiter (\\t)"="," ("delimiter (\\t)")) -> ("error out"=w1663:errorcluster)  [unwired: 8 in, 1 out]
      n755 = Strip Path(path=w1648) -> (name=w1681:string)  [unwired: 1 out]
      n756 = Unbundle(w1682) -> ("DUT"=w1680:string, "Ion (ex Kr)"=w1679:string, "Board Number"=w1678:string, "Effective LET"=w1677:string, "Test Type"=w1676:T22)  [unwired: 1 out]
      n757 = case shown="\"Single Event Latchup\", Default" w1676 {
        tunnel: ["Single Event Latchup (SEL)" "Single Event Transient (SET)"] -> w1675
        frame "Single Event Latchup", Default {
        }
        frame "Single Event Transient" {
        }
      }
      n758 = Build Array("Run Number" ("name"), "DUT" ("element"), "Ion" ("element"), "Board Number" ("element"), "Effective LET" ("element"), "Test Type" ("element")) -> (w1674:string[])
      n759 = Build Array(w1681, w1680, w1679, w1678, w1677, w1675) -> (w1673:string[])
      n760 = Build Array(w1674, w1673) -> (w1662:string[][])
      n761 = Build Path(base path=w1648, name or relative path="RunData_Params.csv") -> (appended path=w1668:path)
      n762 = call-poly <vilib>:"Write Delimited Spreadsheet.vi"("file path (dialog if empty)"=w1668, "format (%s)"="%s" ("format (%.3f)"), "2D data"=w1662, "error in (no error)"=w1663, "transpose? (no:F)"=TRUE, "delimiter (\\t)"="," ("delimiter (\\t)")) -> ("error out"=w1650:errorcluster)  [unwired: 8 in, 1 out]
      n763 = for {
        shift-right: [w1775] -> w1641
        shift-left: w1650 -> [w1774]
        tunnel: string[] ["DCPower", "Oscilloscope"] -> [w1771] mode=indexing
        tunnel: w1648 -> [w1772]
        n764 = Build Path(base path=w1772, name or relative path=w1771) -> (appended path=w1773:path)
        n765 = List Folder(path=w1773, pattern="*NULL.txt", error in=w1774) -> (path out=w1777:path, filenames=w1778:string[], error out=w1779:errorcluster)  [unwired: 1 in, 1 out]
        n766 = for {
          tunnel: [w1780] -> _
          tunnel: w1777 -> [w1780]
          tunnel: w1778 -> [w1782] mode=indexing
          shift-right: [w1783] -> w1775
          shift-left: w1779 -> [w1784]
          n767 = Build Path(base path=w1780, name or relative path=w1782) -> (appended path=w1781:path)
          n768 = Delete(path (use dialog)=w1781, error in=w1784) -> (error out=w1783:errorcluster)  [unwired: 3 in, 2 out]
        }
      }
      n769 = List Folder(path=w1648, error in=w1641) -> (path out=w1646:path, filenames=w1656:string[], folder names=w1647:string[], error out=w1640:errorcluster)  [unwired: 2 in]
      n770 = Strip Path(path=w1648) -> (name=w1658:string)  [unwired: 1 out]
      n771 = Concatenate Strings(w1658, "_OUTPUTS_COPYFOLDER" ("name or relative path")) -> (w1659:string)
      n772 = Build Path(base path=w1648, name or relative path=w1659) -> (appended path=w1655:path)
      n773 = Create Folder(path (use dialog)=w1655, error in=w1640) -> (created path=w1657:path, error out=w1642:errorcluster)  [unwired: 1 in, 1 out]
      n774 = for {
        tunnel: w1646 -> [w1790]
        tunnel: w1656 -> [w1789] mode=indexing
        tunnel: w1657 -> [w1785]
        shift-right: [w1792] -> w1644
        shift-left: w1642 -> [w1786]
        tunnel: [w1785] -> w1645
        n775 = Build Path(base path=w1790, name or relative path=w1789) -> (appended path=w1787:path)
        n776 = Build Path(base path=w1785, name or relative path=w1789) -> (appended path=w1788:path)
        n777 = Copy(8:w1786, 9:TRUE ("overwrite (F)"), 10:w1788, 11:w1787) -> (0:w1792:errorcluster)  [unwired: 1 in, 2 out]
      }
      n778 = for {
        tunnel: w1646 -> [w1768]
        tunnel: w1647 -> [w1767] mode=indexing
        tunnel: w1645 -> [w1763]
        shift-right: [w1770] -> w1643
        shift-left: w1644 -> [w1764]
        tunnel: [w1763] -> _
        n779 = Build Path(base path=w1768, name or relative path=w1767) -> (appended path=w1765:path)
        n780 = Build Path(base path=w1763, name or relative path=w1767) -> (appended path=w1766:path)
        n781 = Copy(8:w1764, 9:TRUE ("overwrite (F)"), 10:w1766, 11:w1765) -> (0:w1770:errorcluster)  [unwired: 1 in, 2 out]
      }
    }
  }
  "Run Data SubPanel Output" <- w155
  "Data Was Collected?" <- w150
  "DCPowerInfoArray" <- w149
  "OscilloscopeInfoArray" <- w137
  "RFSourceInfoArray" <- w145
  "RF Subpanel Output" <- w157
  "error out" <- w138
  "Oscilloscope Info Array" <- w136
  "VISAPowerInfoOutputArray" <- w121
  "DCPowerInformationClusterArray_Output" <- w9
